vi "EC_Applied_Motion_SXSYSZ_20170419A_3chNoBKBACKUP.vi"() -> ()   [LabVIEW 2015]
uses:
  <vilib>/Instr/_visa.llb/VISA Configure Serial Port (Instr).vi
  <userlib>/caLab/Private/Put_DBL-1D_PV-1D.vi
  <userlib>/caLab/Private/Get_PV-1D.vi
  <vilib>/Utility/file.llb/Write To Spreadsheet File (I64).vi
  <vilib>/Utility/file.llb/Read From Spreadsheet File (I64).vi
panel:
  out "APX:FZ_DOWN":dbl
  out "APX:FZ_UP":dbl
  out "APX:FY_DOWN":dbl
  out "APX:FY_UP":dbl
  out "APX:FX_DOWN":dbl
  out "APX:FX_UP":dbl
  out "FZ Jog Counts In Range?":bool
  out "FY Jog Counts In Range?":bool
  out "FX Jog Counts In Range?":bool
  in  "FZ Jog counts":u8
  in  "FY Jog counts":u8
  in  "FX Jog counts":i8
  in  "GFS":bool=TRUE
  out "Isolated from GND?":bool
  in  "Crash Override":bool
  out "Dev5 Voltage 2":dbl
  out "Dev5 Voltage":dbl
  in  "Override":bool
  in  "APX:FZabs":dbl
  in  "Move Z":bool
  in  "Jog Z-":bool
  in  "Jog X-":bool
  in  "Jog Y-":bool
  out "Z Velocity MV mm/sec":dbl format="%.3f"
  out "Z Position MV mm":dbl
  out "Y Velocity MV mm/sec":dbl format="%.3f"
  out "Y Position MV mm":dbl
  out "X Velocity MV mm/sec":dbl format="%.3f"
  out "X Position MV mm":dbl
  in  "stop":bool
  in  "Tab Control 3":enum32{"Status", "Reset"}(tab)
  out "Y in Range":bool
  out "Y in Motion":bool
  out "X  in Range":bool
  out "X  in Motion":bool
  out "Z in Range":bool
  out "Z in Motion":bool
  out "X Ready":bool
  out "Y Ready":bool
  out "Z Ready":bool
  in  "Reset Y Position mm":dbl
  out "Reset Y Motor Steps":i32
  in  "Reset X Position mm":dbl
  out "Reset X Motor Steps":i32
  in  "Reset Z Position mm":dbl
  out "Reset Z Motor Steps":i32
  in  "Reset":bool
  in  "Tab Control":enum32{"mm", "preset", "step"}(tab)
  in  "APX:FXstep":dbl=0.1
  in  "FX Velocity SP mm/sec":dbl=0.01
  in  "APX:FYstep":dbl=0.05
  in  "FY Velocity SP mm/sec":dbl=0.01
  in  "APX:Fzstep":dbl=0.1
  in  "FZ Velocity SP mm/sec":dbl=0.01
  in  "Z Jog Set":bool
  in  "Y Jog Set":bool
  in  "X Jog Set":bool
  in  "X Velocity SP step/sec":i32 min=1 max=1000
  in  "Y Velocity SP step/sec":i32 min=1 max=1000
  in  "Z Velocity SP step/sec":i32 min=1 max=500
  in  "Y Step SP":i32=-20000 min=-800000 max=800000 step=500
  in  "X Step SP":i32=-20000 min=-750000 max=750000 step=500
  in  "Z Step SP":i32=-20000 min=-3000 max=102400000 step=500
  out "X Step PV":i32 max=2000
  out "Y Step PV":i32 max=2000
  out "Z Step PV":i32 max=2000
  out "R Step PV":i32 max=2000
  out "Z COM PORT":refnum<visa-resource-name>="COM5"
  out "Z Holding Current %":i32
  out "Z Run Current %":i32
  out "Z offset mm":dbl
  out "Z mm/rev":dbl
  out "Z steps/rev":u32
  out "Z  velocity PV step/sec":i32
  out "Z MINPOS":i32=-94296
  out "Z MAXPOS":i32=-34296
  in  "Jog Z+":bool
  out "Z Position mm PV":dbl
  out "X Position mm PV":dbl
  out "X velocity PV step/sec":i32
  in  "Jog X+":bool
  out "X Holding Current %":i32
  out "X Run Current %":i32
  out "X offset mm":dbl
  out "X mm/rev":dbl
  out "X steps/rev":u32
  out "X MAXPOS":i32=-34296
  out "X MINPOS":i32=-94296
  out "X COM PORT":refnum<visa-resource-name>="COM5"
  out "Y Holding Current %":i32
  out "Y Run Current %":i32
  out "Y Position mm PV":dbl
  out "Y offset mm":dbl
  out "Y mm/rev":dbl
  out "Y steps/rev":u32
  out "Y velocity PV step/sec":i32
  in  "Stop":bool
  in  "Jog Y+":bool
  out "Y MINPOS":i32=-94296
  out "Y MAXPOS":i32=-34296
  out "Y COM PORT":refnum<visa-resource-name>="COM5"
  # "APX:FY"
  # "x-ray"
  # "APX:FZ"
  # "APX:FX"
  # "SPEAR"
  # "APX:FinePos"
  # "Stage"
  # "Current position"
  # "Jog step/velovity"
  # "sample to SSRL"
  # "FX"
  # "FY"
  # "FZ"
  # "R,L = green"
  # "L"
  # "M"
  # "B"
  # "S"
  # "R"
  # "Preset position"
types:
  T1 = enum16{"Power-up Signature", "Accel Rate", "Accel Max", "Bit Rate", "Buffer Status", "Change Current", "Commence Jogging", "Change Jog Speed", "Continue", "Define Address", "Distance for FC,FM,FO,FY", "Decel Rate", "Distance or Position", "Define Limits", "Encoder Deadband", "Encoder Function", "Encoder Position", "Encoder Ratio", "Feed to Length with Speed Change", "Feed to Length", "Feed to Sensor with Mask Dist", "Feed to Length & Set Output", "Feed to Position", "Feed to Sensor", "Feed to Sensor w/safety", "Follow Handwheel", "Immediate Distance?", "Immediate Encoder?", "Immediate Low Output", "Immediate High Output", "Immediate Position?", "Input Status?", "Jog Accel/Decel", "Jog Disable", "Jog Enable", "Jog Speed", "Motor Disable", "Motor Enable", "Microstep Resolution", "Power up Current", "Power up Mode", "Pause", "Request Status", "Revision Level?", "Seek Home", "Stop Jogging", "Stop & Kill Buffer", "Set Output", "Set ABS Position", "Send String", "Stop", "Velocity for Speed Change", "Velocity Setting", "Wait for Input", "Wait Time"}
  T2 = enum8{"Enabled", "Disabled", "Disabled and Grayed Out"}
  T3 = cluster{"first row[0]":i64, "first row[1]":i64, "first row[2]":i64, "first row[3]":i64, "first row[4]":i64, "first row[5]":i64, "first row[6]":i64, "first row[7]":i64, "first row[8]":i64}
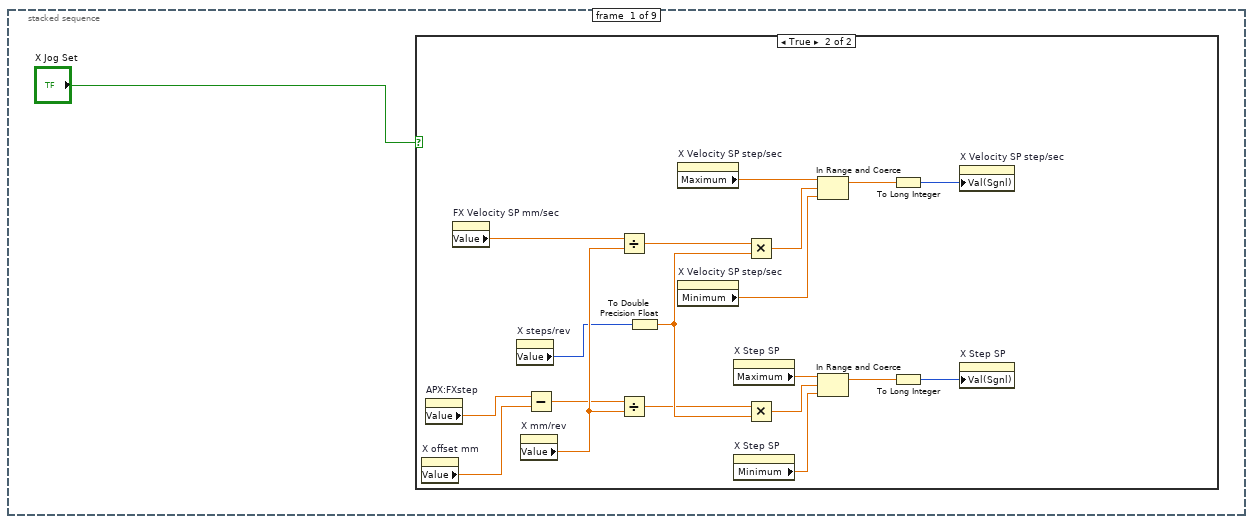
[diagram p5: hidden frame]
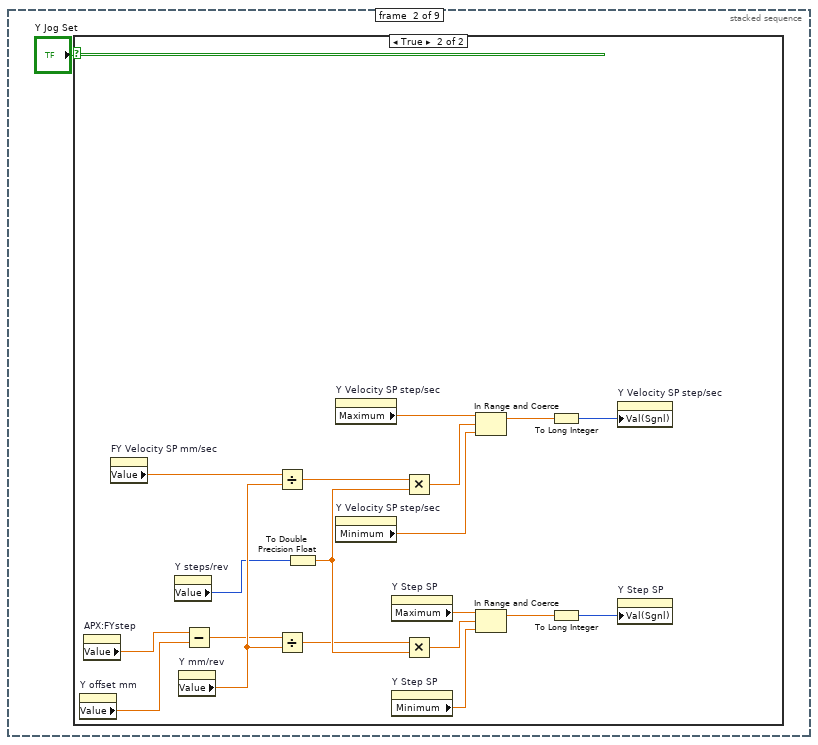
[diagram p7: hidden frame]
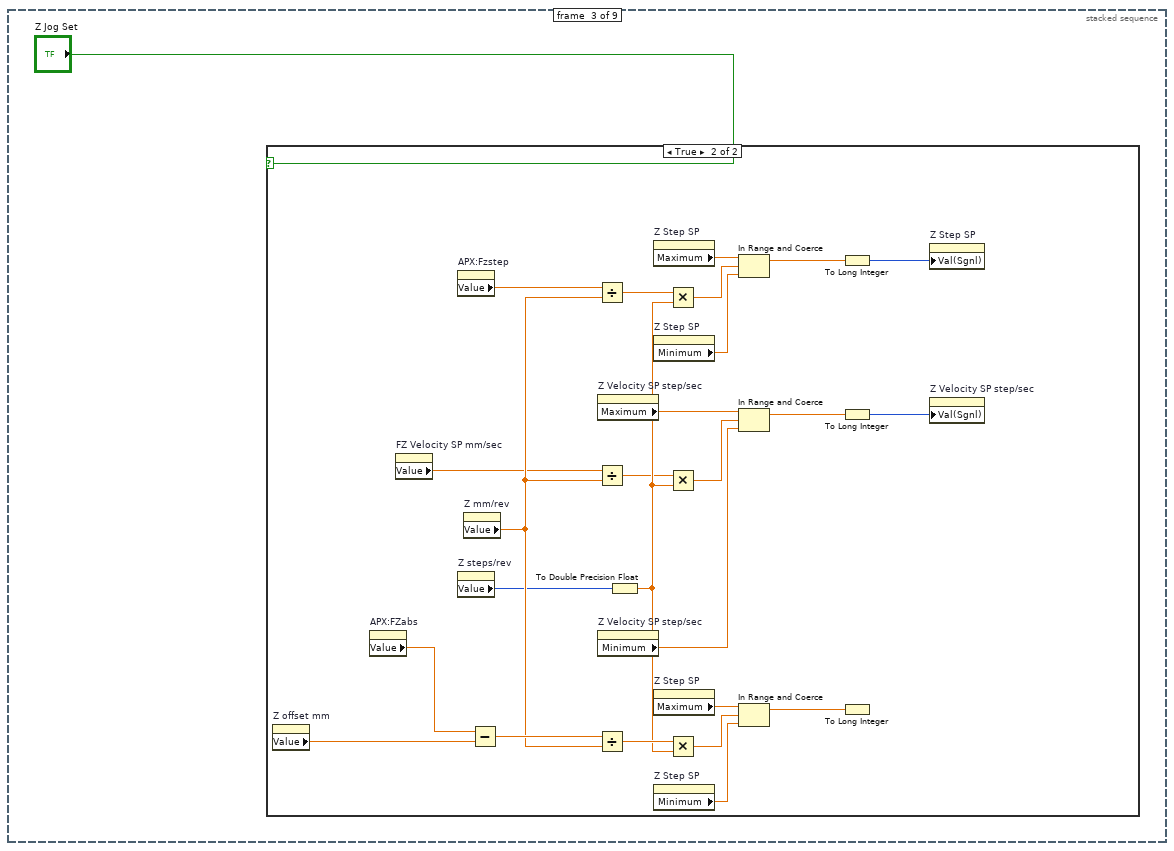
[diagram p9: hidden frame]
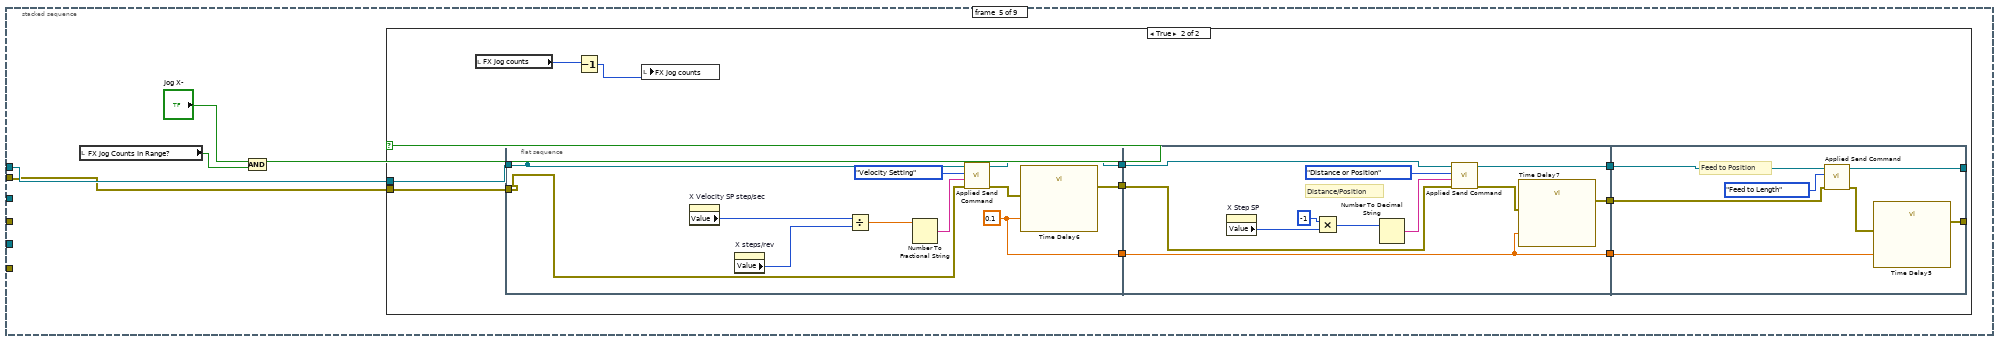
[diagram p12: hidden frame]
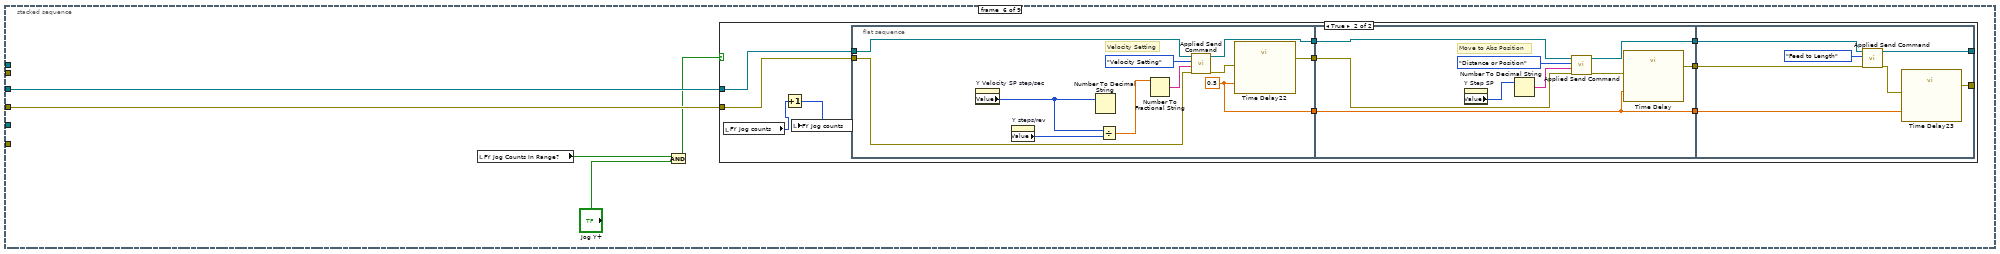
[diagram p14: hidden frame]
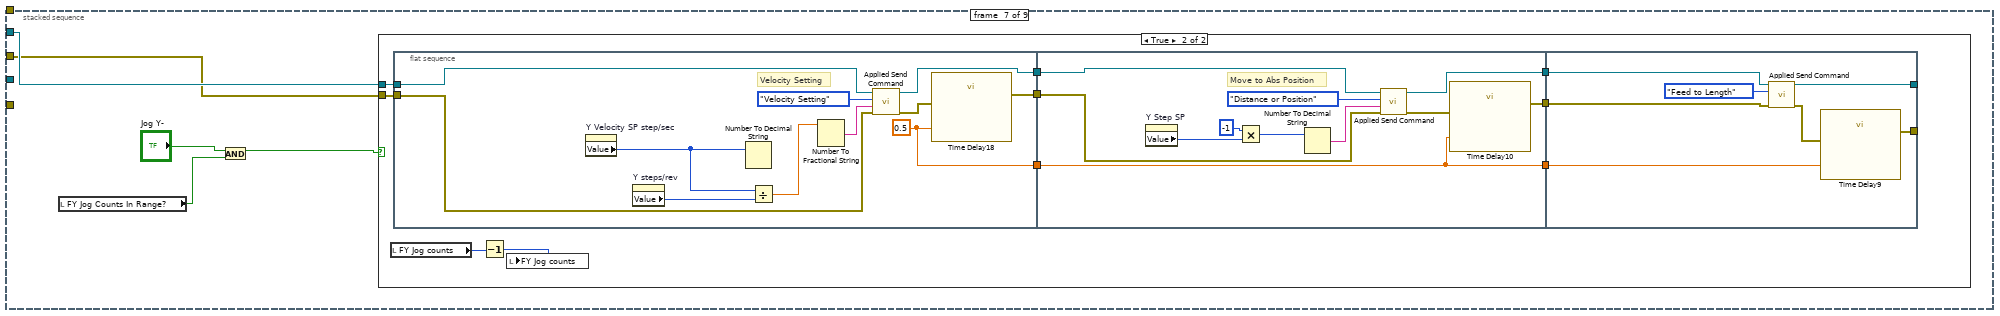
[diagram p16: hidden frame]
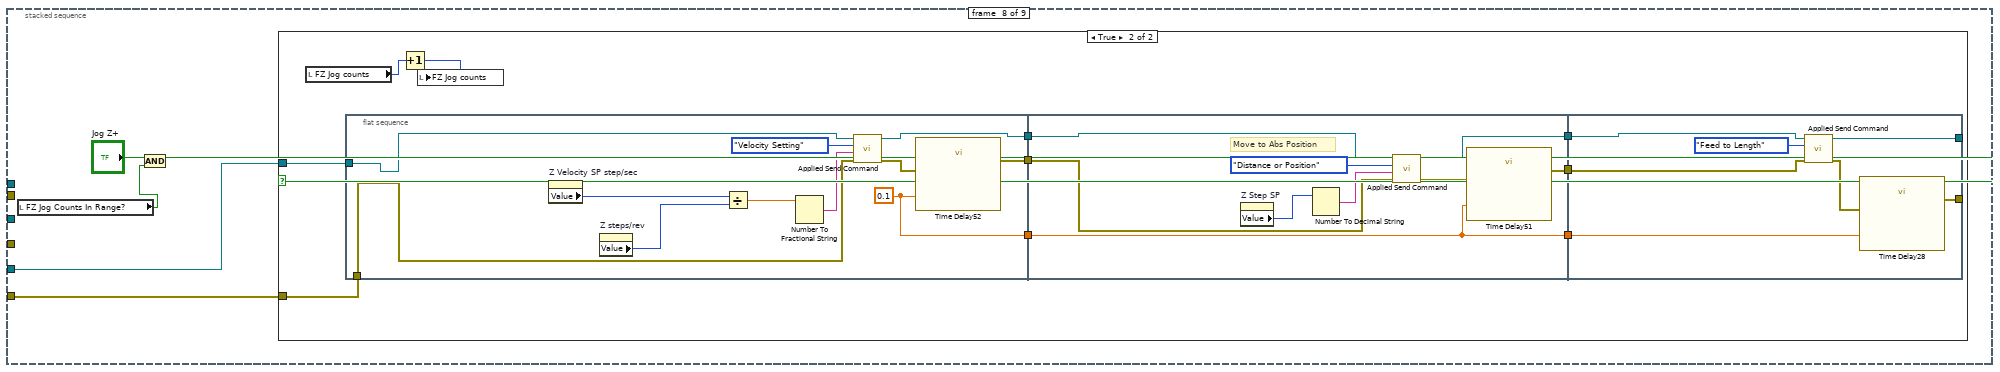
[diagram p18: hidden frame]
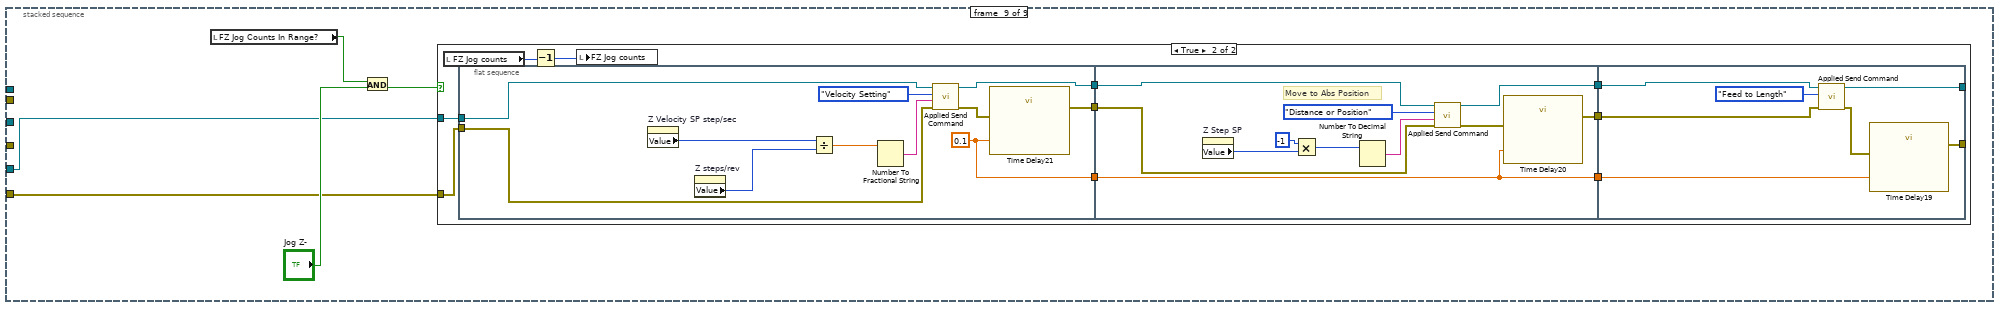
[diagram p20: hidden frame]
diagram:
  (unwired) FALSE
  n1 = flat-sequence {
    tunnel: [w58] -> w18
    tunnel: [w57] -> w17
    tunnel: w18 -> [w75]
    tunnel: w17 -> [w74]
    tunnel: [w73] -> w16
    tunnel: [w72] -> w15
    tunnel: [w78] -> w40
    tunnel: w16 -> [w86]
    tunnel: w15 -> [w85]
    tunnel: [w79] -> w14
    tunnel: w40 -> [w100]
    tunnel: [w99] -> w34
    tunnel: [w97] -> w33
    tunnel: [w102] -> w32
    tunnel: w14 -> [w101]
    tunnel: [w108] -> w38
    tunnel: [w109] -> w39
    tunnel: w34 -> [w109]
    tunnel: w33 -> [w108]
    tunnel: w32 -> [w107]
    frame #0 {
      "X Run Current %" <- 100 ("Run Current %")
      "X Holding Current %" <- 50 ("Holding Current %")
    }
    frame #1 {
      w45 = T2."Enabled" ("Disabled")
      n2 = property on="Jog X+" class="Bool"("DisabledEnum"=w45) -> ()  [unwired: 2 in, 2 out]
      n3 = property on="Jog X-" class="Bool"("DisabledEnum"=w45) -> ()  [unwired: 2 in, 2 out]
      n4 = property on="Jog Y+" class="Bool"("DisabledEnum"=w45) -> ()  [unwired: 2 in, 2 out]
      n5 = property on="Jog Z+" class="Bool"("DisabledEnum"=w45) -> ()  [unwired: 2 in, 2 out]
      n6 = property on="Jog Y-" class="Bool"("DisabledEnum"=w45) -> ()  [unwired: 2 in, 2 out]
      n7 = property on="Jog Z-" class="Bool"("DisabledEnum"=w45) -> ()  [unwired: 2 in, 2 out]
    }
    frame #2 {
      w48 = 0.21167 ("MM/rev")
      w51 = u32 20000 ("step/rev")
      w46 = 1000 ("Value (Signaling)")
      (unwired) 0.01 ("Value (Signaling)")
      n8 = property on="X Velocity SP step/sec" class="DigNum (strict)"("Minimum"=1.0 ("Data Entry Limits:Minimum")) -> ()  [unwired: 2 in, 2 out]
      n9 = property on="X Velocity SP step/sec" class="DigNum (strict)"("Val(Sgnl)"=w46) -> ()  [unwired: 2 in, 2 out]
      n10 = To Double Precision Float(number=w51) -> (double precision float=w50:dbl)
      n11 = To Double Precision Float(number=w46) -> (double precision float=w52:dbl)
      n12 = property on="X Velocity SP step/sec" class="DigNum (strict)"("Maximum"=w52) -> ()  [unwired: 2 in, 2 out]
      n13 = Divide(x=w52, y=w50) -> (x/y=w47:dbl)
      n14 = Multiply(x=w47, y=w48) -> (x*y=w49:dbl)
      n15 = property on="FX Velocity SP mm/sec" class="DigNum (strict)"("Val(Sgnl)"=w49) -> ()  [unwired: 2 in, 2 out]
      "X steps/rev" <- w51
      "X mm/rev" <- w48
    }
    frame #3 {
      w56 = -750000 ("lower limit")
      w55 = 750000 ("upper limit")
      n16 = property on="X Step SP" class="DigNum (strict)"("Maximum"=w55) -> ()  [unwired: 2 in, 2 out]
      n17 = property on="X Step SP" class="DigNum (strict)"("Minimum"=w56) -> ()  [unwired: 2 in, 2 out]
      "X offset mm" <- 0.0 ("offset")
      "X MAXPOS" <- w55
      "X MINPOS" <- w56
    }
    frame #4 {
      w65 = refnum<visa-resource-name> "COM21" ("COM PORT")
      w63 = u16 0 items=["None", "XON/XOFF", "RTS/CTS", "XON/XOFF & RTS/CTS", "DTR/DSR", "XON/XOFF & DTR/DSR"] ("flow control (0:none)")
      w62 = u16 10 items=["1.0"=10, "1.5"=15, "2.0"=20] ("stop bits (10: 1 bit)")
      # "Stop bits"
      n18 = call-poly "VISA Configure Serial Port"("VISA resource name"=w65, "timeout (10sec)"=u32 10000, "baud rate (9600)"=u32 9600, "data bits (8)"=u16 8, "parity (0:none)"=enum16{"None", "Odd", "Even", "Mark", "Space"}."None", "stop bits (10: 1 bit)"=w62, "flow control (0:none)"=w63) -> ("VISA resource name out"=w58:refnum<visa-resource-name>, "error out"=w57:errorcluster)  [unwired: 7 in]
      "X COM PORT" <- w65
    }
    frame #5 {
      n19 = property on="X Run Current" class="DigNum (strict)"() -> ("Value"=w70:i32)  [unwired: 2 in, 2 out]
      n20 = Divide(x=w70, y=100) -> (x/y=w67:dbl)
      n21 = Multiply(x=3.5 ("y"), y=w67) -> (x*y=w69:dbl)
      n22 = Number To Fractional String(number=w69) -> (F-format string=w71:string)  [unwired: 3 in]
      n23 = call "Applied Send Command.vi"("error in (no error)"=w74, "Extra"=w71, "Command"=T1."Change Current", "VISA resource name"=w75) -> ("error out"=w73:errorcluster, "VISA resource name out"=w72:refnum<visa-resource-name>)  [unwired: 3 in, 1 out]
    }
    frame #6 {
      # "VELOCITY"
      n24 = property on="X Velocity SP step/sec" class="DigNum (strict)"() -> ("Value"=w82:i32)  [unwired: 2 in, 2 out]
      n25 = property on="X steps/rev" class="DigNum (strict)"() -> ("Value"=w81:u32)  [unwired: 2 in, 2 out]
      n26 = Divide(x=w82, y=w81) -> (x/y=w80:dbl)
      n27 = Number To Fractional String(number=w80) -> (F-format string=w87:string)  [unwired: 3 in]
      n28 = call "Applied Send Command.vi"("error in (no error)"=w86, "Extra"=w87, "Command"=T1."Velocity Setting", "VISA resource name"=w85) -> ("error out"=w88:errorcluster, "VISA resource name out"=w95:refnum<visa-resource-name>)  [unwired: 3 in, 1 out]
      n29 = call "Time Delay30"("error in (no error)"=w88, "Delay Time (s)"=0.1) -> ("error out"=w93:errorcluster)  [unwired: 9 in]
      n30 = call "Applied Send Command.vi"("error in (no error)"=w93, "Extra"="", "Command"=T1."Velocity Setting", "VISA resource name"=w95) -> ("error out"=w78:errorcluster, "read buffer"=w91:string, "VISA resource name out"=w79:refnum<visa-resource-name>)  [unwired: 3 in]
      n31 = Fract/Exp String To Number(string=w91, offset=3) -> (number=w84:dbl)  [unwired: 2 in, 1 out]
      n32 = Multiply(x=w84, y=w81) -> (x*y=w83:dbl)
      n33 = property on="X velocity PV step/sec" class="DigNum (strict)"("Val(Sgnl)"=w83) -> ()  [unwired: 2 in, 2 out]
    }
    frame #7 {
      # "GET CURRENT POSITION"
      n34 = call "Applied Send Command.vi"("error in (no error)"=w100, "Extra"="", "Command"=T1."Immediate Position?", "VISA resource name"=w101) -> ("error out"=w98:errorcluster, "read buffer"=w104:string, "VISA resource name out"=w99:refnum<visa-resource-name>)  [unwired: 3 in]
      n35 = call "Time Delay13"("error in (no error)"=w98, "Delay Time (s)"=0.1) -> ("error out"=w97:errorcluster)  [unwired: 9 in]
      n36 = Hexadecimal String To Number(string=w104, offset=3) -> (number=w102:u32)  [unwired: 1 in, 1 out]
    }
    frame #8 {
      n37 = disable-structure shown="Disabled" {
        disable-tunnel: w107 -> [w110 _]
        frame Disabled {
          n38 = property on="X Step SP" class="DigNum (strict)"("Val(Sgnl)"=w110) -> ()  [unwired: 2 in, 2 out]
          n39 = property on="X Step SP" class="DigNum (strict)"() -> ("Maximum"=w113:dbl)  [unwired: 2 in, 2 out]
          n40 = property on="X Step SP" class="DigNum (strict)"() -> ("Minimum"=w112:dbl)  [unwired: 2 in, 2 out]
          n41 = In Range and Coerce(upper limit=w113, x=w110, lower limit=w112) -> (In Range?=w111:bool)  [unwired: 1 out]
          n42 = property on="X  in Range" class="Bool (strict)"("Val(Sgnl)"=w111) -> ()  [unwired: 2 in, 2 out]
        }
        frame Enabled {
        }
      }
    }
  }
  n43 = flat-sequence {
    frame #0 {
    }
    frame #1 {
      n44 = call-poly <vilib>:"Read From Spreadsheet File.vi"("file path (dialog if empty)"=path "S:/SSE/SCL2/POS.TXT") -> ("first row"=w114:i64[])  [unwired: 6 in, 4 out]
      n45 = Array To Cluster(array=w114) -> (cluster=w115:T3)
      n46 = Unbundle(w115) -> ("first row[0]"=w117:i64, "first row[1]"=w118:i64, "first row[2]"=w119:i64)  [unwired: 6 out]
      n47 = property on="Reset X Motor Steps" class="DigNum (strict)"("Val(Sgnl)"=w117) -> ()  [unwired: 2 in, 2 out]
      n48 = property on="Reset Y Motor Steps" class="DigNum (strict)"("Val(Sgnl)"=w118) -> ()  [unwired: 2 in, 2 out]
      n49 = property on="Reset Z Motor Steps" class="DigNum (strict)"("Val(Sgnl)"=w119) -> ()  [unwired: 2 in, 2 out]
    }
  }
  n50 = flat-sequence {
    tunnel: [w134] -> w5
    tunnel: [w133] -> w4
    tunnel: w5 -> [w148]
    tunnel: w4 -> [w147]
    tunnel: [w146] -> w3
    tunnel: [w145] -> w2
    tunnel: [w156] -> w31
    tunnel: [w155] -> w30
    tunnel: w3 -> [w158]
    tunnel: w2 -> [w157]
    tunnel: w31 -> [w173]
    tunnel: w30 -> [w172]
    tunnel: [w174] -> w29
    tunnel: [w175] -> w28
    tunnel: [w176] -> w1
    tunnel: [w184] -> w26
    tunnel: [w185] -> w27
    tunnel: w29 -> [w185]
    tunnel: w28 -> [w184]
    tunnel: w1 -> [w183]
    frame #0 {
      "Z Run Current %" <- 100 ("Z Run Current %")
      "Z Holding Current %" <- 50 ("Z Holding Current %")
    }
    frame #1 {
    }
    frame #2 {
      (unwired) 0.05 ("Value (Signaling)")
      w124 = 2.54 ("Z mm/rev")
      w123 = u32 20000 ("step/rev")
      w125 = 500 ("Value (Signaling)")
      n51 = property on="Z Velocity SP step/sec" class="DigNum (strict)"("Minimum"=1.0 ("Data Entry Limits:Minimum")) -> ()  [unwired: 2 in, 2 out]
      n52 = property on="Z Velocity SP step/sec" class="DigNum (strict)"("Val(Sgnl)"=w125) -> ()  [unwired: 2 in, 2 out]
      n53 = To Double Precision Float(number=w123) -> (double precision float=w128:dbl)
      n54 = To Double Precision Float(number=w125) -> (double precision float=w129:dbl)
      n55 = property on="Z Velocity SP step/sec" class="DigNum (strict)"("Maximum"=w129) -> ()  [unwired: 2 in, 2 out]
      n56 = Divide(x=w129, y=w128) -> (x/y=w126:dbl)
      n57 = Multiply(x=w126, y=w124) -> (x*y=w127:dbl)
      n58 = property on="FZ Velocity SP mm/sec" class="DigNum (strict)"("Val(Sgnl)"=w127) -> ()  [unwired: 2 in, 2 out]
      "Z mm/rev" <- w124
      "Z steps/rev" <- w123
    }
    frame #3 {
      w131 = -3000 ("lower limit")
      w130 = 102400000 ("upper limit")
      n59 = property on="Z Step SP" class="DigNum (strict)"("Minimum"=w131) -> ()  [unwired: 2 in, 2 out]
      n60 = property on="Z Step SP" class="DigNum (strict)"("Maximum"=w130) -> ()  [unwired: 2 in, 2 out]
      "Z offset mm" <- 0.0 ("Z offset mm")
      "Z MINPOS" <- w131
      "Z MAXPOS" <- w130
    }
    frame #4 {
      w141 = refnum<visa-resource-name> "COM23" ("COM PORT")
      w139 = u16 0 items=["None", "XON/XOFF", "RTS/CTS", "XON/XOFF & RTS/CTS", "DTR/DSR", "XON/XOFF & DTR/DSR"] ("flow control (0:none)")
      w138 = u16 10 items=["1.0"=10, "1.5"=15, "2.0"=20] ("stop bits (10: 1 bit)")
      # "Stop bits"
      n61 = call-poly "VISA Configure Serial Port"("VISA resource name"=w141, "timeout (10sec)"=u32 10000, "baud rate (9600)"=u32 9600, "data bits (8)"=u16 8, "parity (0:none)"=enum16{"None", "Odd", "Even", "Mark", "Space"}."None", "stop bits (10: 1 bit)"=w138, "flow control (0:none)"=w139) -> ("VISA resource name out"=w134:refnum<visa-resource-name>, "error out"=w133:errorcluster)  [unwired: 7 in]
      "Z COM PORT" <- w141
    }
    frame #5 {
      # "Run Current %"
      n62 = property on="Z Run Current %" class="DigNum (strict)"() -> ("Value"=w149:i32)  [unwired: 2 in, 2 out]
      n63 = Divide(x=w149, y=100) -> (x/y=w150:dbl)
      n64 = Multiply(x=w150, y=3.5) -> (x*y=w144:dbl)
      n65 = Number To Fractional String(number=w144) -> (F-format string=w151:string)  [unwired: 3 in]
      n66 = call "Applied Send Command.vi"("error in (no error)"=w147, "Extra"=w151, "Command"=T1."Change Current", "VISA resource name"=w148) -> ("error out"=w145:errorcluster, "VISA resource name out"=w146:refnum<visa-resource-name>)  [unwired: 3 in, 1 out]
    }
    frame #6 {
      # "VELOCITY"
      n67 = property on="Z Velocity SP step/sec" class="DigNum (strict)"() -> ("Value"=w153:i32)  [unwired: 2 in, 2 out]
      n68 = property on="Z steps/rev" class="DigNum (strict)"() -> ("Value"=w154:u32)  [unwired: 2 in, 2 out]
      n69 = Divide(x=w153, y=w154) -> (x/y=w161:dbl)
      n70 = Number To Fractional String(number=w161) -> (F-format string=w163:string)  [unwired: 3 in]
      n71 = call "Applied Send Command.vi"("error in (no error)"=w157, "Extra"=w163, "Command"=T1."Velocity Setting", "VISA resource name"=w158) -> ("error out"=w164:errorcluster, "VISA resource name out"=w171:refnum<visa-resource-name>)  [unwired: 3 in, 1 out]
      n72 = call "Time Delay2"("error in (no error)"=w164, "Delay Time (s)"=0.1) -> ("error out"=w169:errorcluster)  [unwired: 9 in]
      n73 = call "Applied Send Command.vi"("error in (no error)"=w169, "Extra"="", "Command"=T1."Velocity Setting", "VISA resource name"=w171) -> ("error out"=w155:errorcluster, "read buffer"=w167:string, "VISA resource name out"=w156:refnum<visa-resource-name>)  [unwired: 3 in]
      n74 = Fract/Exp String To Number(string=w167, offset=3) -> (number=w162:dbl)  [unwired: 2 in, 1 out]
      n75 = Multiply(x=w162, y=w154) -> (x*y=w159:dbl)
      n76 = property on="Z  velocity PV step/sec" class="DigNum (strict)"("Val(Sgnl)"=w159) -> ()  [unwired: 2 in, 2 out]
    }
    frame #7 {
      # "GET CURRENT POSITION"
      n77 = call "Applied Send Command.vi"("error in (no error)"=w172, "Extra"="", "Command"=T1."Immediate Position?", "VISA resource name"=w173) -> ("error out"=w178:errorcluster, "read buffer"=w180:string, "VISA resource name out"=w174:refnum<visa-resource-name>)  [unwired: 3 in]
      n78 = call "Time Delay8"("error in (no error)"=w178, "Delay Time (s)"=0.1) -> ("error out"=w175:errorcluster)  [unwired: 9 in]
      n79 = Hexadecimal String To Number(string=w180, offset=3) -> (number=w176:u32)  [unwired: 1 in, 1 out]
    }
    frame #8 {
      n80 = disable-structure shown="Disabled" {
        disable-tunnel: w183 -> [w188 _]
        frame Disabled {
          n81 = property on="Z Step SP" class="DigNum (strict)"("Val(Sgnl)"=w188) -> ()  [unwired: 2 in, 2 out]
          n82 = property on="Z Step SP" class="DigNum (strict)"() -> ("Maximum"=w187:dbl)  [unwired: 2 in, 2 out]
          n83 = property on="Z Step SP" class="DigNum (strict)"() -> ("Minimum"=w186:dbl)  [unwired: 2 in, 2 out]
          n84 = In Range and Coerce(upper limit=w187, x=w188, lower limit=w186) -> (In Range?=w189:bool)  [unwired: 1 out]
          n85 = property on="Z in Range" class="Bool (strict)"("Val(Sgnl)"=w189) -> ()  [unwired: 2 in, 2 out]
        }
        frame Enabled {
        }
      }
    }
  }
  n86 = flat-sequence {
    tunnel: [w204] -> w13
    tunnel: [w203] -> w12
    tunnel: w13 -> [w218]
    tunnel: w12 -> [w217]
    tunnel: [w216] -> w11
    tunnel: [w215] -> w10
    tunnel: w11 -> [w226]
    tunnel: w10 -> [w225]
    tunnel: [w224] -> w9
    tunnel: [w223] -> w8
    tunnel: [w243] -> w35
    tunnel: w9 -> [w246]
    tunnel: w8 -> [w245]
    tunnel: [w244] -> w7
    tunnel: [w242] -> w6
    tunnel: [w253] -> w41
    tunnel: [w255] -> w42
    tunnel: w35 -> [w253]
    tunnel: w7 -> [w255]
    tunnel: w6 -> [w254]
    frame #0 {
      "Y Run Current %" <- 100 ("Run Current %")
      "Y Holding Current %" <- 50 ("Holding Current %")
    }
    frame #1 {
    }
    frame #2 {
      w194 = 0.21167 ("MM/rev")
      w197 = u32 20000 ("step/rev")
      w192 = 1000 ("Value (Signaling)")
      (unwired) 0.01 ("Value (Signaling)")
      n87 = property on="Y Velocity SP step/sec" class="DigNum (strict)"("Minimum"=1.0 ("Data Entry Limits:Minimum")) -> ()  [unwired: 2 in, 2 out]
      n88 = property on="Y Velocity SP step/sec" class="DigNum (strict)"("Val(Sgnl)"=w192) -> ()  [unwired: 2 in, 2 out]
      n89 = To Double Precision Float(number=w197) -> (double precision float=w196:dbl)
      n90 = To Double Precision Float(number=w192) -> (double precision float=w198:dbl)
      n91 = property on="Y Velocity SP step/sec" class="DigNum (strict)"("Maximum"=w198) -> ()  [unwired: 2 in, 2 out]
      n92 = Divide(x=w198, y=w196) -> (x/y=w193:dbl)
      n93 = Multiply(x=w193, y=w194) -> (x*y=w195:dbl)
      n94 = property on="FY Velocity SP mm/sec" class="DigNum (strict)"("Val(Sgnl)"=w195) -> ()  [unwired: 2 in, 2 out]
      "Y steps/rev" <- w197
      "Y mm/rev" <- w194
    }
    frame #3 {
      w201 = -800000 ("lower limit")
      w202 = 800000 ("upper limit")
      n95 = property on="Y Step SP" class="DigNum (strict)"("Maximum"=w202) -> ()  [unwired: 2 in, 2 out]
      n96 = property on="Y Step SP" class="DigNum (strict)"("Minimum"=w201) -> ()  [unwired: 2 in, 2 out]
      "Y MAXPOS" <- w202
      "Y MINPOS" <- w201
      "Y offset mm" <- 0.0 ("offset")
    }
    frame #4 {
      w211 = refnum<visa-resource-name> "COM22" ("COM PORT")
      w209 = u16 0 items=["None", "XON/XOFF", "RTS/CTS", "XON/XOFF & RTS/CTS", "DTR/DSR", "XON/XOFF & DTR/DSR"] ("flow control (0:none)")
      w208 = u16 10 items=["1.0"=10, "1.5"=15, "2.0"=20] ("stop bits (10: 1 bit)")
      # "Stop bits"
      n97 = call-poly "VISA Configure Serial Port"("VISA resource name"=w211, "timeout (10sec)"=u32 10000, "baud rate (9600)"=u32 9600, "data bits (8)"=u16 8, "parity (0:none)"=enum16{"None", "Odd", "Even", "Mark", "Space"}."None", "stop bits (10: 1 bit)"=w208, "flow control (0:none)"=w209) -> ("VISA resource name out"=w204:refnum<visa-resource-name>, "error out"=w203:errorcluster)  [unwired: 7 in]
      "Y COM PORT" <- w211
    }
    frame #5 {
      n98 = property on="Y Run Current %" class="DigNum (strict)"() -> ("Value"=w219:i32)  [unwired: 2 in, 2 out]
      n99 = Divide(x=w219, y=100) -> (x/y=w220:dbl)
      n100 = Multiply(x=w220, y=3.5) -> (x*y=w214:dbl)
      n101 = Number To Fractional String(number=w214) -> (F-format string=w221:string)  [unwired: 3 in]
      n102 = call "Applied Send Command.vi"("error in (no error)"=w217, "Extra"=w221, "Command"=T1."Change Current", "VISA resource name"=w218) -> ("error out"=w215:errorcluster, "VISA resource name out"=w216:refnum<visa-resource-name>)  [unwired: 3 in, 1 out]
    }
    frame #6 {
      # "VELOCITY"
      n103 = property on="Y Velocity SP step/sec" class="DigNum (strict)"() -> ("Value"=w227:i32)  [unwired: 2 in, 2 out]
      n104 = property on="Y steps/rev" class="DigNum (strict)"() -> ("Value"=w230:u32)  [unwired: 2 in, 2 out]
      n105 = Divide(x=w227, y=w230) -> (x/y=w229:dbl)
      n106 = Number To Fractional String(number=w229) -> (F-format string=w233:string)  [unwired: 3 in]
      n107 = call "Applied Send Command.vi"("error in (no error)"=w225, "Extra"=w233, "Command"=T1."Velocity Setting", "VISA resource name"=w226) -> ("error out"=w234:errorcluster, "VISA resource name out"=w241:refnum<visa-resource-name>)  [unwired: 3 in, 1 out]
      n108 = call "Time Delay36"("error in (no error)"=w234, "Delay Time (s)"=0.1) -> ("error out"=w239:errorcluster)  [unwired: 9 in]
      n109 = call "Applied Send Command.vi"("error in (no error)"=w239, "Extra"="", "Command"=T1."Velocity Setting", "VISA resource name"=w241) -> ("error out"=w223:errorcluster, "read buffer"=w237:string, "VISA resource name out"=w224:refnum<visa-resource-name>)  [unwired: 3 in]
      n110 = Fract/Exp String To Number(string=w237, offset=3) -> (number=w232:dbl)  [unwired: 2 in, 1 out]
      n111 = Multiply(x=w232, y=w230) -> (x*y=w231:dbl)
      n112 = property on="Y velocity PV step/sec" class="DigNum (strict)"("Val(Sgnl)"=w231) -> ()  [unwired: 2 in, 2 out]
    }
    frame #7 {
      # "GET CURRENT POSITION"
      n113 = call "Applied Send Command.vi"("error in (no error)"=w245, "Extra"="", "Command"=T1."Immediate Position?", "VISA resource name"=w246) -> ("error out"=w248:errorcluster, "read buffer"=w250:string, "VISA resource name out"=w244:refnum<visa-resource-name>)  [unwired: 3 in]
      n114 = call "Time Delay37"("error in (no error)"=w248, "Delay Time (s)"=0.1) -> ("error out"=w243:errorcluster)  [unwired: 9 in]
      n115 = Hexadecimal String To Number(string=w250, offset=3) -> (number=w242:u32)  [unwired: 1 in, 1 out]
    }
    frame #8 {
      n116 = disable-structure shown="Disabled" {
        disable-tunnel: w254 -> [w258 _]
        frame Disabled {
          n117 = property on="Y Step SP" class="DigNum (strict)"("Val(Sgnl)"=w258) -> ()  [unwired: 2 in, 2 out]
          n118 = property on="Y Step SP" class="DigNum (strict)"() -> ("Maximum"=w257:dbl)  [unwired: 2 in, 2 out]
          n119 = property on="Y Step SP" class="DigNum (strict)"() -> ("Minimum"=w256:dbl)  [unwired: 2 in, 2 out]
          n120 = In Range and Coerce(upper limit=w257, x=w258, lower limit=w256) -> (In Range?=w259:bool)  [unwired: 1 out]
          n121 = property on="Y in Range" class="Bool (strict)"("Val(Sgnl)"=w259) -> ()  [unwired: 2 in, 2 out]
        }
        frame Enabled {
        }
      }
    }
  }
  n122 = while {
    tunnel: w42 -> [w275]
    tunnel: w41 -> [w274]
    tunnel: [w295] -> w22
    tunnel: [w294] -> w23
    tunnel: w39 -> [w277]
    tunnel: w38 -> [w276]
    tunnel: [w292] -> w37
    tunnel: [w291] -> w36
    tunnel: w27 -> [w273]
    tunnel: w26 -> [w272]
    tunnel: [w290] -> w25
    tunnel: [w289] -> w24
    tunnel: [w288] -> _
    tunnel: [w287] -> _
    stop <- "stop" stop-if-true
    n123 = flat-sequence {
      frame #0 {
      }
      frame #1 {
      }
    }
    n124 = flat-sequence {
      frame #0 {
      }
      frame #1 {
      }
    }
    n125 = local read "X Position mm PV"() -> (w284:dbl)
    n126 = local read "Y Position mm PV"() -> (w283:dbl)
    n127 = local read "Z Position mm PV"() -> (w285:dbl)
    n128 = local read "FZ Jog counts"() -> (w261:u8)
    n129 = local read "FY Jog counts"() -> (w265:u8)
    n130 = local read "FX Jog counts"() -> (w269:i8)
    n131 = Build Array("APX:PiezeX", "APX:PiezeY", "APX:PiezeZ") -> (w279:string[])
    n132 = Build Array(w284, w283, w285) -> (w278:dbl[])
    n133 = flat-sequence {
      frame #0 {
        n134 = disable-structure shown="Disabled" {
          frame Disabled {
            w662 = 10 ("number of samples")
            n135 = call "DAQ Assistant"("number of samples"=w662) -> ("data"=w667:dynamicdata)  [unwired: 16 in, 2 out]
            n136 = call "Convert from Dynamic Data"("Dynamic Data Type"=w667) -> ("Array"=w668:dbl[])  [unwired: 3 in]
            n137 = Add Array Elements(numeric array=w668) -> (sum=w666:dbl)
            n138 = Divide(x=w666, y=w662) -> (x/y=w665:dbl)
            n139 = Absolute Value(x=w665) -> (abs(x)=w669:dbl)
            "Dev5 Voltage" <- w669
            n140 = Multiply(x=0.5, y=0.8) -> (x*y=w663:dbl)
            n141 = Greater?(x=w669, y=w663) -> (0:w670:bool)
            n142 = case shown="True" "Override" {
              tunnel: [w672 TRUE] -> _
              tunnel: w670 -> [w672 _]
              frame False {
              }
              frame True {
              }
            }
          }
          frame Enabled {
          }
        }
      }
    }
    n143 = call-poly <userlib>:"CaLabPut.vi"("Values"=w278, "PV Names"=w279) -> ()  [unwired: 6 in, 4 out]
    n144 = In Range and Coerce(upper limit=10.0, x=w269, lower limit=-10.0) -> (In Range?=→"FX Jog Counts In Range?":bool)  [unwired: 1 out]
    n145 = In Range and Coerce(upper limit=4.0, x=w265, lower limit=-4.0) -> (In Range?=→"FY Jog Counts In Range?":bool)  [unwired: 1 out]
    n146 = In Range and Coerce(upper limit=20.0, x=w261, lower limit=-2.0) -> (In Range?=→"FZ Jog Counts In Range?":bool)  [unwired: 1 out]
    n147 = flat-sequence {
      frame #0 {
        w304 = 0 ("index (col)")
        w311 = 0.0 ("element")
        n148 = Build Array("APX:FX_UP", "APX:FX_DOWN", "APX:FY_UP", "APX:FY_DOWN", "APX:FZ_UP", "APX:FZ_DOWN") -> (w312:string[])
        n149 = call-poly "CaLabGet.vi"("PV Names"=w312) -> ("Value Array (number)"=w302:dbl[][])  [unwired: 8 in, 6 out]
        n150 = Build Array(w311, w311, w311, w311, w311, w311) -> (w310:dbl[])
        n151 = call-poly <userlib>:"CaLabPut.vi"("Values"=w310, "PV Names"=w312) -> ()  [unwired: 6 in, 4 out]
        n152 = Index Array(array=w302, index (row)=0 ("disabled index (row)"), index (col)=w304) -> (element=→"APX:FX_UP":dbl)
        n153 = Index Array(array=w302, index (row)=1, index (col)=w304) -> (element=→"APX:FX_DOWN":dbl)
        n154 = Index Array(array=w302, index (row)=4, index (col)=w304) -> (element=→"APX:FZ_UP":dbl)
        n155 = Index Array(array=w302, index (row)=2, index (col)=w304) -> (element=→"APX:FY_UP":dbl)
        n156 = Index Array(array=w302, index (row)=5, index (col)=w304) -> (element=→"APX:FZ_DOWN":dbl)
        n157 = Index Array(array=w302, index (row)=3, index (col)=w304) -> (element=→"APX:FY_DOWN":dbl)
      }
    }
    n158 = stacked-sequence {
      tunnel: w277 -> [_ _ _ w388 w430 _ _ _ _]
      tunnel: w276 -> [_ _ _ w387 w429 _ _ _ _]
      tunnel: w275 -> [_ _ _ _ _ w474 w517 _ _]
      tunnel: w274 -> [_ _ _ _ _ w473 w516 _ _]
      tunnel: w273 -> [_ _ _ _ _ _ _ w560 w602]
      tunnel: w272 -> [_ _ _ _ _ _ _ w559 w601]
      frame #0 {
        n159 = case shown="True" "X Jog Set" {
          frame False {
          }
          frame True {
            n160 = property on="X offset mm" class="DigNum (strict)"() -> ("Value"=w324:dbl)  [unwired: 2 in, 2 out]
            n161 = property on="APX:FXstep" class="DigNum (strict)"() -> ("Value"=w325:dbl)  [unwired: 2 in, 2 out]
            n162 = property on="FX Velocity SP mm/sec" class="DigNum (strict)"() -> ("Value"=w331:dbl)  [unwired: 2 in, 2 out]
            n163 = property on="X steps/rev" class="DigNum (strict)"() -> ("Value"=w322:u32)  [unwired: 2 in, 2 out]
            n164 = property on="X mm/rev" class="DigNum (strict)"() -> ("Value"=w338:dbl)  [unwired: 2 in, 2 out]
            n165 = Subtract(x=w325, y=w324) -> (x-y=w321:dbl)
            n166 = Divide(x=w331, y=w338) -> (x/y=w330:dbl)
            n167 = Divide(x=w321, y=w338) -> (x/y=w320:dbl)
            n168 = To Double Precision Float(number=w322) -> (double precision float=w337:dbl)
            n169 = property on="X Velocity SP step/sec" class="DigNum (strict)"() -> ("Maximum"=w335:dbl)  [unwired: 2 in, 2 out]
            n170 = property on="X Velocity SP step/sec" class="DigNum (strict)"() -> ("Minimum"=w336:dbl)  [unwired: 2 in, 2 out]
            n171 = property on="X Step SP" class="DigNum (strict)"() -> ("Maximum"=w328:dbl)  [unwired: 2 in, 2 out]
            n172 = property on="X Step SP" class="DigNum (strict)"() -> ("Minimum"=w329:dbl)  [unwired: 2 in, 2 out]
            n173 = Multiply(x=w330, y=w337) -> (x*y=w333:dbl)
            n174 = Multiply(x=w320, y=w337) -> (x*y=w326:dbl)
            n175 = In Range and Coerce(upper limit=w335, x=w333, lower limit=w336) -> (coerced(x)=w334:dbl)  [unwired: 1 out]
            n176 = In Range and Coerce(upper limit=w328, x=w326, lower limit=w329) -> (coerced(x)=w327:dbl)  [unwired: 1 out]
            n177 = To Long Integer(number=w334) -> (32bit integer=w332:i32)
            n178 = To Long Integer(number=w327) -> (32bit integer=w323:i32)
            n179 = property on="X Velocity SP step/sec" class="DigNum (strict)"("Val(Sgnl)"=w332) -> ()  [unwired: 2 in, 2 out]
            n180 = property on="X Step SP" class="DigNum (strict)"("Val(Sgnl)"=w323) -> ()  [unwired: 2 in, 2 out]
          }
        }
      }
      frame #1 {
        n181 = case shown="True" "Y Jog Set" {
          frame False {
          }
          frame True {
            n182 = property on="Y offset mm" class="DigNum (strict)"() -> ("Value"=w344:dbl)  [unwired: 2 in, 2 out]
            n183 = property on="APX:FYstep" class="DigNum (strict)"() -> ("Value"=w345:dbl)  [unwired: 2 in, 2 out]
            n184 = property on="FY Velocity SP mm/sec" class="DigNum (strict)"() -> ("Value"=w351:dbl)  [unwired: 2 in, 2 out]
            n185 = property on="Y steps/rev" class="DigNum (strict)"() -> ("Value"=w342:u32)  [unwired: 2 in, 2 out]
            n186 = property on="Y mm/rev" class="DigNum (strict)"() -> ("Value"=w358:dbl)  [unwired: 2 in, 2 out]
            n187 = Subtract(x=w345, y=w344) -> (x-y=w341:dbl)
            n188 = Divide(x=w351, y=w358) -> (x/y=w350:dbl)
            n189 = Divide(x=w341, y=w358) -> (x/y=w340:dbl)
            n190 = To Double Precision Float(number=w342) -> (double precision float=w357:dbl)
            n191 = property on="Y Velocity SP step/sec" class="DigNum (strict)"() -> ("Maximum"=w355:dbl)  [unwired: 2 in, 2 out]
            n192 = property on="Y Velocity SP step/sec" class="DigNum (strict)"() -> ("Minimum"=w356:dbl)  [unwired: 2 in, 2 out]
            n193 = property on="Y Step SP" class="DigNum (strict)"() -> ("Maximum"=w348:dbl)  [unwired: 2 in, 2 out]
            n194 = property on="Y Step SP" class="DigNum (strict)"() -> ("Minimum"=w349:dbl)  [unwired: 2 in, 2 out]
            n195 = Multiply(x=w350, y=w357) -> (x*y=w353:dbl)
            n196 = Multiply(x=w340, y=w357) -> (x*y=w346:dbl)
            n197 = In Range and Coerce(upper limit=w355, x=w353, lower limit=w356) -> (coerced(x)=w354:dbl)  [unwired: 1 out]
            n198 = In Range and Coerce(upper limit=w348, x=w346, lower limit=w349) -> (coerced(x)=w347:dbl)  [unwired: 1 out]
            n199 = To Long Integer(number=w354) -> (32bit integer=w352:i32)
            n200 = To Long Integer(number=w347) -> (32bit integer=w343:i32)
            n201 = property on="Y Velocity SP step/sec" class="DigNum (strict)"("Val(Sgnl)"=w352) -> ()  [unwired: 2 in, 2 out]
            n202 = property on="Y Step SP" class="DigNum (strict)"("Val(Sgnl)"=w343) -> ()  [unwired: 2 in, 2 out]
          }
        }
      }
      frame #2 {
        n203 = case shown="True" "Z Jog Set" {
          frame False {
          }
          frame True {
            n204 = property on="Z offset mm" class="DigNum (strict)"() -> ("Value"=w382:dbl)  [unwired: 2 in, 2 out]
            n205 = property on="APX:FZabs" class="DigNum (strict)"() -> ("Value"=w384:dbl)  [unwired: 2 in, 2 out]
            n206 = property on="FZ Velocity SP mm/sec" class="DigNum (strict)"() -> ("Value"=w369:dbl)  [unwired: 2 in, 2 out]
            n207 = property on="APX:Fzstep" class="DigNum (strict)"() -> ("Value"=w363:dbl)  [unwired: 2 in, 2 out]
            n208 = property on="Z steps/rev" class="DigNum (strict)"() -> ("Value"=w361:u32)  [unwired: 2 in, 2 out]
            n209 = property on="Z mm/rev" class="DigNum (strict)"() -> ("Value"=w381:dbl)  [unwired: 2 in, 2 out]
            n210 = Subtract(x=w384, y=w382) -> (x-y=w383:dbl)
            n211 = Divide(x=w363, y=w381) -> (x/y=w360:dbl)
            n212 = Divide(x=w369, y=w381) -> (x/y=w368:dbl)
            n213 = Divide(x=w383, y=w381) -> (x/y=w380:dbl)
            n214 = property on="Z Velocity SP step/sec" class="DigNum (strict)"() -> ("Maximum"=w373:dbl)  [unwired: 2 in, 2 out]
            n215 = property on="Z Velocity SP step/sec" class="DigNum (strict)"() -> ("Minimum"=w374:dbl)  [unwired: 2 in, 2 out]
            n216 = To Double Precision Float(number=w361) -> (double precision float=w379:dbl)
            n217 = property on="Z Step SP" class="DigNum (strict)"() -> ("Maximum"=w366:dbl)  [unwired: 2 in, 2 out]
            n218 = property on="Z Step SP" class="DigNum (strict)"() -> ("Minimum"=w367:dbl)  [unwired: 2 in, 2 out]
            n219 = property on="Z Step SP" class="DigNum (strict)"() -> ("Maximum"=w376:dbl)  [unwired: 2 in, 2 out]
            n220 = property on="Z Step SP" class="DigNum (strict)"() -> ("Minimum"=w377:dbl)  [unwired: 2 in, 2 out]
            n221 = Multiply(x=w360, y=w379) -> (x*y=w364:dbl)
            n222 = Multiply(x=w368, y=w379) -> (x*y=w371:dbl)
            n223 = Multiply(x=w380, y=w379) -> (x*y=w378:dbl)
            n224 = In Range and Coerce(upper limit=w366, x=w364, lower limit=w367) -> (coerced(x)=w365:dbl)  [unwired: 1 out]
            n225 = In Range and Coerce(upper limit=w373, x=w371, lower limit=w374) -> (coerced(x)=w372:dbl)  [unwired: 1 out]
            n226 = In Range and Coerce(upper limit=w376, x=w378, lower limit=w377) -> (coerced(x)=w375:dbl)  [unwired: 1 out]
            n227 = To Long Integer(number=w365) -> (32bit integer=w362:i32)
            n228 = To Long Integer(number=w372) -> (32bit integer=w370:i32)
            n229 = To Long Integer(number=w375) -> ()  [unwired: 1 out]
            n230 = property on="Z Step SP" class="DigNum (strict)"("Val(Sgnl)"=w362) -> ()  [unwired: 2 in, 2 out]
            n231 = property on="Z Velocity SP step/sec" class="DigNum (strict)"("Val(Sgnl)"=w370) -> ()  [unwired: 2 in, 2 out]
          }
        }
      }
      frame #3 {
        n232 = local read "FX Jog Counts In Range?"() -> (w385:bool)
        n233 = And(x="Jog X+", y=w385) -> (x .and. y?=w386:bool)
        n234 = case shown="True" w386 {
          tunnel: w388 -> [_ w393]
          tunnel: w387 -> [_ w392]
          frame False {
          }
          frame True {
            n235 = flat-sequence {
              tunnel: [w404] -> w399
              tunnel: [w401] -> w398
              tunnel: [w400] -> w397
              tunnel: w393 -> [w406]
              tunnel: w392 -> [w405]
              tunnel: w399 -> [w413]
              tunnel: [w412] -> w396
              tunnel: w398 -> [w414]
              tunnel: [w415] -> w395
              tunnel: w397 -> [w411]
              tunnel: [w411] -> w394
              tunnel: w396 -> [w426]
              tunnel: w395 -> [w425]
              tunnel: [w424] -> _
              tunnel: [w423] -> _
              tunnel: w394 -> [w422]
              frame #0 {
                w400 = 0.1 ("Delay Time (s)")
                n236 = property on="X Velocity SP step/sec" class="DigNum (strict)"() -> ("Value"=w403:i32)  [unwired: 2 in, 2 out]
                n237 = property on="X steps/rev" class="DigNum (strict)"() -> ("Value"=w407:u32)  [unwired: 2 in, 2 out]
                n238 = Divide(x=w403, y=w407) -> (x/y=w408:dbl)
                n239 = Number To Fractional String(number=w408) -> (F-format string=w409:string)  [unwired: 3 in]
                n240 = call "Applied Send Command.vi"("error in (no error)"=w405, "Extra"=w409, "Command"=T1."Velocity Setting", "VISA resource name"=w406) -> ("error out"=w402:errorcluster, "VISA resource name out"=w404:refnum<visa-resource-name>)  [unwired: 3 in, 1 out]
                n241 = call "Time Delay14"("error in (no error)"=w402, "Delay Time (s)"=w400) -> ("error out"=w401:errorcluster)  [unwired: 9 in]
              }
              frame #1 {
                # "Distance/Position"
                n242 = property on="X Step SP" class="DigNum (strict)"() -> ("Value"=w416:i32)  [unwired: 2 in, 2 out]
                n243 = Number To Decimal String(number=w416) -> (decimal integer string=w418:string)  [unwired: 1 in]
                n244 = call "Applied Send Command.vi"("error in (no error)"=w414, "Extra"=w418, "Command"=T1."Distance or Position", "VISA resource name"=w413) -> ("error out"=w417:errorcluster, "VISA resource name out"=w412:refnum<visa-resource-name>)  [unwired: 3 in, 1 out]
                n245 = call "Time Delay31"("error in (no error)"=w417, "Delay Time (s)"=w411) -> ("error out"=w415:errorcluster)  [unwired: 9 in]
              }
              frame #2 {
                # "Feed to Position"
                n246 = call "Applied Send Command.vi"("error in (no error)"=w425, "Command"=T1."Feed to Length", "VISA resource name"=w426) -> ("error out"=w420:errorcluster, "VISA resource name out"=w424:refnum<visa-resource-name>)  [unwired: 4 in, 1 out]
                n247 = call "Time Delay15"("error in (no error)"=w420, "Delay Time (s)"=w422) -> ("error out"=w423:errorcluster)  [unwired: 9 in]
              }
            }
            n248 = local read "FX Jog counts"() -> (w391:i8)
            n249 = Increment(x=w391) -> (x+1=w390:i8)
            n250 = local write "FX Jog counts"(w390) -> ()
          }
        }
      }
      frame #4 {
        n251 = local read "FX Jog Counts In Range?"() -> (w427:bool)
        n252 = And(x="Jog X-", y=w427) -> (x .and. y?=w428:bool)
        n253 = case shown="True" w428 {
          tunnel: w430 -> [_ w435]
          tunnel: w429 -> [_ w434]
          frame False {
          }
          frame True {
            n254 = local read "FX Jog counts"() -> (w433:i8)
            n255 = flat-sequence {
              tunnel: [w448] -> w441
              tunnel: [w445] -> w440
              tunnel: [w444] -> w439
              tunnel: [w443] -> _
              tunnel: w435 -> [w443]
              tunnel: w434 -> [w442]
              tunnel: w441 -> [w457]
              tunnel: [w456] -> w438
              tunnel: w440 -> [w458]
              tunnel: [w459] -> w437
              tunnel: w439 -> [w455]
              tunnel: [w455] -> w436
              tunnel: w438 -> [w470]
              tunnel: w437 -> [w469]
              tunnel: [w468] -> _
              tunnel: [w467] -> _
              tunnel: w436 -> [w466]
              frame #0 {
                w444 = 0.1 ("Delay Time (s)")
                n256 = property on="X Velocity SP step/sec" class="DigNum (strict)"() -> ("Value"=w447:i32)  [unwired: 2 in, 2 out]
                n257 = property on="X steps/rev" class="DigNum (strict)"() -> ("Value"=w449:u32)  [unwired: 2 in, 2 out]
                n258 = Divide(x=w447, y=w449) -> (x/y=w450:dbl)
                n259 = Number To Fractional String(number=w450) -> (F-format string=w451:string)  [unwired: 3 in]
                n260 = call "Applied Send Command.vi"("error in (no error)"=w442, "Extra"=w451, "Command"=T1."Velocity Setting", "VISA resource name"=w443) -> ("error out"=w446:errorcluster, "VISA resource name out"=w448:refnum<visa-resource-name>)  [unwired: 3 in, 1 out]
                n261 = call "Time Delay6"("error in (no error)"=w446, "Delay Time (s)"=w444) -> ("error out"=w445:errorcluster)  [unwired: 9 in]
              }
              frame #1 {
                # "Distance/Position"
                n262 = property on="X Step SP" class="DigNum (strict)"() -> ("Value"=w460:i32)  [unwired: 2 in, 2 out]
                n263 = Multiply(x=-1, y=w460) -> (x*y=w454:i32)
                n264 = Number To Decimal String(number=w454) -> (decimal integer string=w462:string)  [unwired: 1 in]
                n265 = call "Applied Send Command.vi"("error in (no error)"=w458, "Extra"=w462, "Command"=T1."Distance or Position", "VISA resource name"=w457) -> ("error out"=w461:errorcluster, "VISA resource name out"=w456:refnum<visa-resource-name>)  [unwired: 3 in, 1 out]
                n266 = call "Time Delay7"("error in (no error)"=w461, "Delay Time (s)"=w455) -> ("error out"=w459:errorcluster)  [unwired: 9 in]
              }
              frame #2 {
                # "Feed to Position"
                n267 = call "Applied Send Command.vi"("error in (no error)"=w469, "Command"=T1."Feed to Length", "VISA resource name"=w470) -> ("error out"=w464:errorcluster, "VISA resource name out"=w468:refnum<visa-resource-name>)  [unwired: 4 in, 1 out]
                n268 = call "Time Delay5"("error in (no error)"=w464, "Delay Time (s)"=w466) -> ("error out"=w467:errorcluster)  [unwired: 9 in]
              }
            }
            n269 = Decrement(x=w433) -> (x-1=w432:i8)
            n270 = local write "FX Jog counts"(w432) -> ()
          }
        }
      }
      frame #5 {
        n271 = local read "FY Jog Counts In Range?"() -> (w471:bool)
        n272 = And(x=w471, y="Jog Y+") -> (x .and. y?=w472:bool)
        n273 = case shown="True" w472 {
          tunnel: w474 -> [_ w479]
          tunnel: w473 -> [_ w478]
          frame False {
          }
          frame True {
            n274 = local read "FY Jog counts"() -> (w477:u8)
            n275 = Increment(x=w477) -> (x+1=w476:u8)
            n276 = local write "FY Jog counts"(w476) -> ()
            n277 = flat-sequence {
              tunnel: [w492] -> w485
              tunnel: [w487] -> w484
              tunnel: [w486] -> w483
              tunnel: w478 -> [w491]
              tunnel: w479 -> [w490]
              tunnel: [w503] -> w482
              tunnel: [w498] -> w481
              tunnel: w485 -> [w501]
              tunnel: w484 -> [w502]
              tunnel: w483 -> [w499]
              tunnel: [w499] -> w480
              tunnel: [w508] -> _
              tunnel: [w511] -> _
              tunnel: w482 -> [w510]
              tunnel: w481 -> [w509]
              tunnel: w480 -> [w512]
              frame #0 {
                w486 = 0.5 ("Delay Time (s)")
                # "Velocity Setting"
                n278 = property on="Y Velocity SP step/sec" class="DigNum (strict)"() -> ("Value"=w495:i32)  [unwired: 2 in, 2 out]
                n279 = property on="Y steps/rev" class="DigNum (strict)"() -> ("Value"=w494:u32)  [unwired: 2 in, 2 out]
                n280 = Number To Decimal String(number=w495) -> ()  [unwired: 1 in, 1 out]
                n281 = Divide(x=w495, y=w494) -> (x/y=w496:dbl)
                n282 = Number To Fractional String(number=w496) -> (F-format string=w489:string)  [unwired: 3 in]
                n283 = call "Applied Send Command.vi"("error in (no error)"=w491, "Extra"=w489, "Command"=T1."Velocity Setting", "VISA resource name"=w490) -> ("error out"=w488:errorcluster, "VISA resource name out"=w492:refnum<visa-resource-name>)  [unwired: 3 in, 1 out]
                n284 = call "Time Delay22"("error in (no error)"=w488, "Delay Time (s)"=w486) -> ("error out"=w487:errorcluster)  [unwired: 9 in]
              }
              frame #1 {
                # "Move to Abs Position"
                n285 = property on="Y Step SP" class="DigNum (strict)"() -> ("Value"=w505:i32)  [unwired: 2 in, 2 out]
                n286 = Number To Decimal String(number=w505) -> (decimal integer string=w500:string)  [unwired: 1 in]
                n287 = call "Applied Send Command.vi"("error in (no error)"=w502, "Extra"=w500, "Command"=T1."Distance or Position", "VISA resource name"=w501) -> ("error out"=w497:errorcluster, "VISA resource name out"=w503:refnum<visa-resource-name>)  [unwired: 3 in, 1 out]
                n288 = call "Time Delay"("error in (no error)"=w497, "Delay Time (s)"=w499) -> ("error out"=w498:errorcluster)  [unwired: 9 in]
              }
              frame #2 {
                n289 = call "Applied Send Command.vi"("error in (no error)"=w509, "Command"=T1."Feed to Length", "VISA resource name"=w510) -> ("error out"=w506:errorcluster, "VISA resource name out"=w511:refnum<visa-resource-name>)  [unwired: 4 in, 1 out]
                n290 = call "Time Delay23"("error in (no error)"=w506, "Delay Time (s)"=w512) -> ("error out"=w508:errorcluster)  [unwired: 9 in]
              }
            }
          }
        }
      }
      frame #6 {
        n291 = local read "FY Jog Counts In Range?"() -> (w513:bool)
        n292 = And(x="Jog Y-", y=w513) -> (x .and. y?=w514:bool)
        n293 = case shown="True" w514 {
          tunnel: w517 -> [_ w521]
          tunnel: w516 -> [_ w520]
          frame False {
          }
          frame True {
            n294 = local read "FY Jog counts"() -> (w519:u8)
            n295 = flat-sequence {
              tunnel: [w534] -> w527
              tunnel: [w529] -> w526
              tunnel: [w528] -> w525
              tunnel: w520 -> [w533]
              tunnel: w521 -> [w532]
              tunnel: [w547] -> w524
              tunnel: [w542] -> w523
              tunnel: w527 -> [w545]
              tunnel: w526 -> [w546]
              tunnel: w525 -> [w543]
              tunnel: [w543] -> w522
              tunnel: [w552] -> _
              tunnel: [w555] -> _
              tunnel: w524 -> [w554]
              tunnel: w523 -> [w553]
              tunnel: w522 -> [w556]
              frame #0 {
                w528 = 0.5 ("Delay Time (s)")
                # "Velocity Setting"
                n296 = property on="Y Velocity SP step/sec" class="DigNum (strict)"() -> ("Value"=w537:i32)  [unwired: 2 in, 2 out]
                n297 = property on="Y steps/rev" class="DigNum (strict)"() -> ("Value"=w536:u32)  [unwired: 2 in, 2 out]
                n298 = Number To Decimal String(number=w537) -> ()  [unwired: 1 in, 1 out]
                n299 = Divide(x=w537, y=w536) -> (x/y=w538:dbl)
                n300 = Number To Fractional String(number=w538) -> (F-format string=w531:string)  [unwired: 3 in]
                n301 = call "Applied Send Command.vi"("error in (no error)"=w533, "Extra"=w531, "Command"=T1."Velocity Setting", "VISA resource name"=w532) -> ("error out"=w530:errorcluster, "VISA resource name out"=w534:refnum<visa-resource-name>)  [unwired: 3 in, 1 out]
                n302 = call "Time Delay18"("error in (no error)"=w530, "Delay Time (s)"=w528) -> ("error out"=w529:errorcluster)  [unwired: 9 in]
              }
              frame #1 {
                # "Move to Abs Position"
                n303 = property on="Y Step SP" class="DigNum (strict)"() -> ("Value"=w549:i32)  [unwired: 2 in, 2 out]
                n304 = Multiply(x=-1, y=w549) -> (x*y=w540:i32)
                n305 = Number To Decimal String(number=w540) -> (decimal integer string=w544:string)  [unwired: 1 in]
                n306 = call "Applied Send Command.vi"("error in (no error)"=w546, "Extra"=w544, "Command"=T1."Distance or Position", "VISA resource name"=w545) -> ("error out"=w541:errorcluster, "VISA resource name out"=w547:refnum<visa-resource-name>)  [unwired: 3 in, 1 out]
                n307 = call "Time Delay10"("error in (no error)"=w541, "Delay Time (s)"=w543) -> ("error out"=w542:errorcluster)  [unwired: 9 in]
              }
              frame #2 {
                n308 = call "Applied Send Command.vi"("error in (no error)"=w553, "Command"=T1."Feed to Length", "VISA resource name"=w554) -> ("error out"=w550:errorcluster, "VISA resource name out"=w555:refnum<visa-resource-name>)  [unwired: 4 in, 1 out]
                n309 = call "Time Delay9"("error in (no error)"=w550, "Delay Time (s)"=w556) -> ("error out"=w552:errorcluster)  [unwired: 9 in]
              }
            }
            n310 = Decrement(x=w519) -> (x-1=w518:u8)
            n311 = local write "FY Jog counts"(w518) -> ()
          }
        }
      }
      frame #7 {
        n312 = local read "FZ Jog Counts In Range?"() -> (w557:bool)
        n313 = And(x="Jog Z+", y=w557) -> (x .and. y?=w558:bool)
        n314 = case shown="True" w558 {
          tunnel: w560 -> [_ w565]
          tunnel: w559 -> [_ w564]
          frame False {
          }
          frame True {
            n315 = local read "FZ Jog counts"() -> (w563:u8)
            n316 = flat-sequence {
              tunnel: [w577] -> w571
              tunnel: [w575] -> w570
              tunnel: [w574] -> w569
              tunnel: w565 -> [w573]
              tunnel: w564 -> [w572]
              tunnel: [w586] -> w568
              tunnel: [w585] -> w567
              tunnel: w571 -> [w587]
              tunnel: w570 -> [w589]
              tunnel: w569 -> [w583]
              tunnel: [w583] -> w566
              tunnel: [w598] -> _
              tunnel: [w595] -> _
              tunnel: w568 -> [w596]
              tunnel: w567 -> [w594]
              tunnel: w566 -> [w597]
              frame #0 {
                w574 = 0.1 ("Delay Time (s)")
                n317 = property on="Z Velocity SP step/sec" class="DigNum (strict)"() -> ("Value"=w579:i32)  [unwired: 2 in, 2 out]
                n318 = property on="Z steps/rev" class="DigNum (strict)"() -> ("Value"=w578:u32)  [unwired: 2 in, 2 out]
                n319 = Divide(x=w579, y=w578) -> (x/y=w580:dbl)
                n320 = Number To Fractional String(number=w580) -> (F-format string=w581:string)  [unwired: 3 in]
                n321 = call "Applied Send Command.vi"("error in (no error)"=w572, "Extra"=w581, "Command"=T1."Velocity Setting", "VISA resource name"=w573) -> ("error out"=w576:errorcluster, "VISA resource name out"=w577:refnum<visa-resource-name>)  [unwired: 3 in, 1 out]
                n322 = call "Time Delay52"("error in (no error)"=w576, "Delay Time (s)"=w574) -> ("error out"=w575:errorcluster)  [unwired: 9 in]
              }
              frame #1 {
                # "Move to Abs Position"
                n323 = property on="Z Step SP" class="DigNum (strict)"() -> ("Value"=w591:i32)  [unwired: 2 in, 2 out]
                n324 = Number To Decimal String(number=w591) -> (decimal integer string=w588:string)  [unwired: 1 in]
                n325 = call "Applied Send Command.vi"("error in (no error)"=w589, "Extra"=w588, "Command"=T1."Distance or Position", "VISA resource name"=w587) -> ("error out"=w584:errorcluster, "VISA resource name out"=w586:refnum<visa-resource-name>)  [unwired: 3 in, 1 out]
                n326 = call "Time Delay51"("error in (no error)"=w584, "Delay Time (s)"=w583) -> ("error out"=w585:errorcluster)  [unwired: 9 in]
              }
              frame #2 {
                n327 = call "Applied Send Command.vi"("error in (no error)"=w594, "Command"=T1."Feed to Length", "VISA resource name"=w596) -> ("error out"=w592:errorcluster, "VISA resource name out"=w595:refnum<visa-resource-name>)  [unwired: 4 in, 1 out]
                n328 = call "Time Delay28"("error in (no error)"=w592, "Delay Time (s)"=w597) -> ("error out"=w598:errorcluster)  [unwired: 9 in]
              }
            }
            n329 = Increment(x=w563) -> (x+1=w562:u8)
            n330 = local write "FZ Jog counts"(w562) -> ()
          }
        }
      }
      frame #8 {
        n331 = local read "FZ Jog Counts In Range?"() -> (w599:bool)
        n332 = And(x=w599, y="Jog Z-") -> (x .and. y?=w600:bool)
        n333 = case shown="True" w600 {
          tunnel: w602 -> [_ w607]
          tunnel: w601 -> [_ w606]
          frame False {
          }
          frame True {
            n334 = local read "FZ Jog counts"() -> (w605:u8)
            n335 = flat-sequence {
              tunnel: [w617] -> w613
              tunnel: [w615] -> w612
              tunnel: [w614] -> w611
              tunnel: w606 -> [w618]
              tunnel: w607 -> [w619]
              tunnel: [w630] -> w610
              tunnel: [w629] -> w609
              tunnel: w613 -> [w631]
              tunnel: w612 -> [w633]
              tunnel: w611 -> [w627]
              tunnel: [w627] -> w608
              tunnel: [w642] -> _
              tunnel: [w639] -> _
              tunnel: w610 -> [w640]
              tunnel: w609 -> [w638]
              tunnel: w608 -> [w641]
              frame #0 {
                w614 = 0.1 ("Delay Time (s)")
                n336 = property on="Z Velocity SP step/sec" class="DigNum (strict)"() -> ("Value"=w621:i32)  [unwired: 2 in, 2 out]
                n337 = property on="Z steps/rev" class="DigNum (strict)"() -> ("Value"=w620:u32)  [unwired: 2 in, 2 out]
                n338 = Divide(x=w621, y=w620) -> (x/y=w622:dbl)
                n339 = Number To Fractional String(number=w622) -> (F-format string=w623:string)  [unwired: 3 in]
                n340 = call "Applied Send Command.vi"("error in (no error)"=w618, "Extra"=w623, "Command"=T1."Velocity Setting", "VISA resource name"=w619) -> ("error out"=w616:errorcluster, "VISA resource name out"=w617:refnum<visa-resource-name>)  [unwired: 3 in, 1 out]
                n341 = call "Time Delay21"("error in (no error)"=w616, "Delay Time (s)"=w614) -> ("error out"=w615:errorcluster)  [unwired: 9 in]
              }
              frame #1 {
                # "Move to Abs Position"
                n342 = property on="Z Step SP" class="DigNum (strict)"() -> ("Value"=w635:i32)  [unwired: 2 in, 2 out]
                n343 = Multiply(x=-1, y=w635) -> (x*y=w626:i32)
                n344 = Number To Decimal String(number=w626) -> (decimal integer string=w632:string)  [unwired: 1 in]
                n345 = call "Applied Send Command.vi"("error in (no error)"=w633, "Extra"=w632, "Command"=T1."Distance or Position", "VISA resource name"=w631) -> ("error out"=w628:errorcluster, "VISA resource name out"=w630:refnum<visa-resource-name>)  [unwired: 3 in, 1 out]
                n346 = call "Time Delay20"("error in (no error)"=w628, "Delay Time (s)"=w627) -> ("error out"=w629:errorcluster)  [unwired: 9 in]
              }
              frame #2 {
                n347 = call "Applied Send Command.vi"("error in (no error)"=w638, "Command"=T1."Feed to Length", "VISA resource name"=w640) -> ("error out"=w636:errorcluster, "VISA resource name out"=w639:refnum<visa-resource-name>)  [unwired: 4 in, 1 out]
                n348 = call "Time Delay19"("error in (no error)"=w636, "Delay Time (s)"=w641) -> ("error out"=w642:errorcluster)  [unwired: 9 in]
              }
            }
            n349 = Decrement(x=w605) -> (x-1=w604:u8)
            n350 = local write "FZ Jog counts"(w604) -> ()
          }
        }
      }
    }
    n351 = event shown="[0] Timeout" {
      selector: _ -> [_ _ _ _ _ _]
      dyn-events: _ -> [_ _ _ _ _ _]
      timeout: 1 -> [_ _ _ _ _ _]
      tunnel: w274 -> [w735 _ _ w973 w985 w1012]
      tunnel: [_ _ _ w973 w983 w1010] -> w295
      tunnel: w275 -> [w707 _ _ w974 w986 w1013]
      tunnel: [_ _ _ w974 w984 w1011] -> w294
      tunnel: w277 -> [w706 _ _ _ w980 w1009]
      tunnel: w276 -> [w718 _ _ _ w979 w1008]
      tunnel: [_ _ _ _ w982 w1007] -> w292
      tunnel: [_ _ _ _ w981 w1006] -> w291
      tunnel: w273 -> [w708 _ _ _ w978 w1005]
      tunnel: w272 -> [w709 _ _ _ w977 w1004]
      tunnel: [_ _ _ _ w976 _] -> w290
      tunnel: [_ _ _ _ w975 _] -> w289
      tunnel: [_ _ _ _ _ w1003] -> w288
      tunnel: [_ _ _ _ _ w1002] -> w287
      event Timeout {
        n352 = event-data() -> ()  [unwired: 1 in, 2 out]
        n353 = flat-sequence {
          tunnel: [w747] -> w717
          tunnel: [w760] -> w716
          tunnel: [w769] -> w715
          tunnel: [w740] -> w714
          tunnel: w708 -> [w755]
          tunnel: w709 -> [w756]
          tunnel: [w738] -> w675
          tunnel: w717 -> [w779]
          tunnel: [w779] -> w713
          tunnel: w716 -> [w778]
          tunnel: [w778] -> w712
          tunnel: w715 -> [w777]
          tunnel: [w775] -> w711
          tunnel: w714 -> [w776]
          tunnel: [w776] -> w710
          tunnel: w713 -> [w782]
          tunnel: w712 -> [w783]
          tunnel: w711 -> [w781]
          tunnel: w710 -> [w780]
          tunnel: [w780] -> w683
          frame #0 {
            w759 = 0.5 ("Delay Time (s)")
            n354 = call "Applied Send Command.vi"("error in (no error)"=w756, "Command"=T1."Immediate Position?", "VISA resource name"=w755) -> ("error out"=w754:errorcluster, "read buffer"=w751:string, "VISA resource name out"=w749:refnum<visa-resource-name>)  [unwired: 4 in]
            n355 = Hexadecimal String To Number(string=w751, offset=3) -> (number=w752:u32)  [unwired: 1 in, 1 out]
            n356 = property on="Z Step SP" class="DigNum (strict)"() -> ("Maximum"=w771:dbl)  [unwired: 2 in, 2 out]
            n357 = property on="Z Step SP" class="DigNum (strict)"() -> ("Minimum"=w773:dbl)  [unwired: 2 in, 2 out]
            n358 = To Long Integer(number=w752) -> (32bit integer=w761:i32)
            n359 = property on="Z steps/rev" class="DigNum (strict)"() -> ("Value"=w767:u32)  [unwired: 2 in, 2 out]
            n360 = property on="Z Step PV" class="DigNum (strict)"("Val(Sgnl)"=w761) -> ()  [unwired: 2 in, 2 out]
            n361 = To Long Integer(number=w771) -> (32bit integer=w770:i32)
            n362 = To Long Integer(number=w773) -> (32bit integer=w772:i32)
            n363 = In Range and Coerce(upper limit=w770, x=w761, lower limit=w772) -> (In Range?=w769:bool)  [unwired: 1 out]
            n364 = To Double Precision Float(number=w761) -> (double precision float=w762:dbl)
            n365 = To Double Precision Float(number=w767) -> (double precision float=w768:dbl)
            n366 = property on="Z in Range" class="Bool (strict)"("Val(Sgnl)"=w769) -> ()  [unwired: 2 in, 2 out]
            n367 = Divide(x=w762, y=w768) -> (x/y=w766:dbl)
            n368 = call "Time Delay17"("error in (no error)"=w754, "Delay Time (s)"=w759) -> ("error out"=w739:errorcluster)  [unwired: 9 in]
            n369 = property on="Z mm/rev" class="DigNum (strict)"() -> ("Value"=w765:dbl)  [unwired: 2 in, 2 out]
            n370 = property on="Z offset mm" class="DigNum (strict)"() -> ("Value"=w763:dbl)  [unwired: 2 in, 2 out]
            n371 = Multiply(x=w766, y=w765) -> (x*y=w764:dbl)
            n372 = call "Applied Send Command.vi"("error in (no error)"=w739, "Command"=T1."Request Status", "VISA resource name"=w749) -> ("error out"=w748:errorcluster, "read buffer"=w744:string, "VISA resource name out"=w747:refnum<visa-resource-name>)  [unwired: 4 in]
            n373 = call "Time Delay16"("error in (no error)"=w748, "Delay Time (s)"=w759) -> ("error out"=w760:errorcluster)  [unwired: 9 in]
            n374 = Add(x=w764, y=w763) -> (x+y=w738:dbl)
            n375 = String Subset(string=w744, offset (0)=0, length (rest)=1 ("length (rest)")) -> (substring=w741:string)
            n376 = property on="Z Position mm PV" class="DigNum (strict)"("Val(Sgnl)"=w738) -> ()  [unwired: 2 in, 2 out]
            n377 = Equal?(x=w741, y="R") -> (x = y?=w758:bool)
            n378 = Not Equal?(x=w741, y="R") -> (x != y?=w740:bool)
            n379 = property on="Z Ready" class="Bool (strict)"("Val(Sgnl)"=w758) -> ()  [unwired: 2 in, 2 out]
            n380 = property on="Z in Motion" class="Bool (strict)"("Val(Sgnl)"=w740) -> ()  [unwired: 2 in, 2 out]
          }
          frame #1 {
            n381 = local read "Isolated from GND?"() -> (w774:bool)
            n382 = Or(x=w774, y=w777) -> (x .or. y?=w775:bool)
          }
          frame #2 {
            n383 = case shown="False" w781 {
              tunnel: w782 -> [w787 w790]
              tunnel: [w785 w790] -> _
              tunnel: [w784 w789] -> _
              tunnel: w783 -> [w786 w789]
              frame False {
                n384 = call "Applied Send Command.vi"("error in (no error)"=w786, "Command"=T1."Stop & Kill Buffer", "VISA resource name"=w787) -> ("error out"=w784:errorcluster, "VISA resource name out"=w785:refnum<visa-resource-name>)  [unwired: 4 in, 1 out]
              }
              frame True {
              }
            }
          }
        }
        n385 = property on="Y Step SP" class="DigNum (strict)"() -> ("Maximum"=w703:dbl)  [unwired: 2 in, 2 out]
        n386 = property on="Y Step SP" class="DigNum (strict)"() -> ("Minimum"=w702:dbl)  [unwired: 2 in, 2 out]
        n387 = property on="X Step SP" class="DigNum (strict)"() -> ("Maximum"=w698:dbl)  [unwired: 2 in, 2 out]
        n388 = property on="X Step SP" class="DigNum (strict)"() -> ("Minimum"=w699:dbl)  [unwired: 2 in, 2 out]
        n389 = Subtract(x=w703, y=w702) -> (x-y=w704:dbl)
        n390 = Subtract(x=w698, y=w699) -> (x-y=w700:dbl)
        n391 = property on="X Step PV" class="DigNum (strict)"() -> ("Value"=w697:i32)  [unwired: 2 in, 2 out]
        n392 = property on="Y Step PV" class="DigNum (strict)"() -> ("Value"=w696:i32)  [unwired: 2 in, 2 out]
        n393 = Divide(x=w704, y=2.0) -> (x/y=w692:dbl)
        n394 = Divide(x=w700, y=2.0) -> (x/y=w693:dbl)
        n395 = Absolute Value(x=w697) -> (abs(x)=w694:i32)
        n396 = Absolute Value(x=w696) -> (abs(x)=w695:i32)
        n397 = Absolute Value(x=w692) -> (abs(x)=w690:dbl)
        n398 = Absolute Value(x=w693) -> (abs(x)=w691:dbl)
        n399 = Multiply(x=w694, y=w695) -> (x*y=w689:i32)
        n400 = Multiply(x=w690, y=w691) -> (x*y=w688:dbl)
        n401 = Less Or Equal?(x=w689, y=w688) -> (x <= y?=w687:bool)
        n402 = flat-sequence {
          tunnel: w735 -> [w863]
          tunnel: w707 -> [w864]
          tunnel: [w860] -> w734
          tunnel: [w870] -> w732
          tunnel: [w849] -> w730
          tunnel: [w851] -> w728
          tunnel: w703 -> [w850]
          tunnel: w702 -> [w847]
          tunnel: w687 -> [w848]
          tunnel: [w846] -> w676
          tunnel: w734 -> [w889]
          tunnel: [w889] -> w733
          tunnel: w732 -> [w888]
          tunnel: [w888] -> w731
          tunnel: w730 -> [w887]
          tunnel: [w885] -> w729
          tunnel: w728 -> [w886]
          tunnel: [w886] -> w727
          tunnel: w733 -> [w892]
          tunnel: w731 -> [w893]
          tunnel: w729 -> [w891]
          tunnel: w727 -> [w890]
          tunnel: [w890] -> w684
          frame #0 {
            w869 = 0.5 ("Delay Time (s)")
            n403 = call "Applied Send Command.vi"("error in (no error)"=w863, "Command"=T1."Immediate Position?", "VISA resource name"=w864) -> ("error out"=w866:errorcluster, "read buffer"=w867:string, "VISA resource name out"=w861:refnum<visa-resource-name>)  [unwired: 4 in]
            n404 = To Long Integer(number=w850) -> (32bit integer=w881:i32)
            n405 = To Long Integer(number=w847) -> (32bit integer=w882:i32)
            n406 = Hexadecimal String To Number(string=w867, offset=3) -> (number=w871:u32)  [unwired: 1 in, 1 out]
            n407 = To Long Integer(number=w871) -> (32bit integer=w872:i32)
            n408 = property on="Y steps/rev" class="DigNum (strict)"() -> ("Value"=w878:u32)  [unwired: 2 in, 2 out]
            n409 = property on="Y Step PV" class="DigNum (strict)"("Val(Sgnl)"=w872) -> ()  [unwired: 2 in, 2 out]
            n410 = In Range and Coerce(upper limit=w881, x=w872, lower limit=w882) -> (In Range?=w880:bool)  [unwired: 1 out]
            n411 = To Double Precision Float(number=w872) -> (double precision float=w873:dbl)
            n412 = To Double Precision Float(number=w878) -> (double precision float=w879:dbl)
            n413 = Divide(x=w873, y=w879) -> (x/y=w877:dbl)
            n414 = And(x=w880, y=w848) -> (x .and. y?=w849:bool)
            n415 = property on="Y in Range" class="Bool (strict)"("Val(Sgnl)"=w849) -> ()  [unwired: 2 in, 2 out]
            n416 = call "Time Delay4"("error in (no error)"=w866, "Delay Time (s)"=w869) -> ("error out"=w859:errorcluster)  [unwired: 9 in]
            n417 = property on="Y mm/rev" class="DigNum (strict)"() -> ("Value"=w876:dbl)  [unwired: 2 in, 2 out]
            n418 = property on="Y offset mm" class="DigNum (strict)"() -> ("Value"=w874:dbl)  [unwired: 2 in, 2 out]
            n419 = Multiply(x=w877, y=w876) -> (x*y=w875:dbl)
            n420 = call "Applied Send Command.vi"("error in (no error)"=w859, "Command"=T1."Request Status", "VISA resource name"=w861) -> ("error out"=w858:errorcluster, "read buffer"=w855:string, "VISA resource name out"=w860:refnum<visa-resource-name>)  [unwired: 4 in]
            n421 = call "Time Delay3"("error in (no error)"=w858, "Delay Time (s)"=w869) -> ("error out"=w870:errorcluster)  [unwired: 9 in]
            n422 = Add(x=w875, y=w874) -> (x+y=w846:dbl)
            n423 = String Subset(string=w855, offset (0)=0, length (rest)=1 ("length (rest)")) -> (substring=w853:string)
            n424 = property on="Y Position mm PV" class="DigNum (strict)"("Val(Sgnl)"=w846) -> ()  [unwired: 2 in, 2 out]
            n425 = Equal?(x=w853, y="R") -> (x = y?=w868:bool)
            n426 = Not Equal?(x=w853, y="R") -> (x != y?=w851:bool)
            n427 = property on="Y Ready" class="Bool (strict)"("Val(Sgnl)"=w868) -> ()  [unwired: 2 in, 2 out]
            n428 = property on="Y in Motion" class="Bool (strict)"("Val(Sgnl)"=w851) -> ()  [unwired: 2 in, 2 out]
          }
          frame #1 {
            n429 = local read "Isolated from GND?"() -> (w884:bool)
            n430 = Or(x=w887, y=w884) -> (x .or. y?=w885:bool)
          }
          frame #2 {
            n431 = case shown="False" w891 {
              tunnel: w892 -> [w895 w900]
              tunnel: [w897 w900] -> _
              tunnel: [w896 w899] -> _
              tunnel: w893 -> [w894 w899]
              frame False {
                n432 = call "Applied Send Command.vi"("error in (no error)"=w894, "Command"=T1."Stop & Kill Buffer", "VISA resource name"=w895) -> ("error out"=w896:errorcluster, "VISA resource name out"=w897:refnum<visa-resource-name>)  [unwired: 4 in, 1 out]
              }
              frame True {
              }
            }
          }
        }
        n433 = flat-sequence {
          tunnel: [w804] -> w726
          tunnel: [w815] -> w725
          tunnel: [w793] -> w724
          tunnel: [w800] -> w723
          tunnel: w706 -> [w811]
          tunnel: w718 -> [w799]
          tunnel: w698 -> [w795]
          tunnel: w699 -> [w794]
          tunnel: w687 -> [w792]
          tunnel: [w791] -> w677
          tunnel: w726 -> [w834]
          tunnel: [w834] -> w722
          tunnel: w725 -> [w833]
          tunnel: [w833] -> w721
          tunnel: w724 -> [w830]
          tunnel: [w829] -> w720
          tunnel: w723 -> [w832]
          tunnel: [w832] -> w719
          tunnel: w722 -> [w838]
          tunnel: w721 -> [w837]
          tunnel: w720 -> [w836]
          tunnel: w719 -> [w835]
          tunnel: [w835] -> w685
          frame #0 {
            w814 = 0.5 ("Delay Time (s)")
            n434 = To Long Integer(number=w794) -> (32bit integer=w827:i32)
            n435 = To Long Integer(number=w795) -> (32bit integer=w826:i32)
            n436 = call "Applied Send Command.vi"("error in (no error)"=w799, "Command"=T1."Immediate Position?", "VISA resource name"=w811) -> ("error out"=w809:errorcluster, "read buffer"=w810:string, "VISA resource name out"=w805:refnum<visa-resource-name>)  [unwired: 4 in]
            n437 = Hexadecimal String To Number(string=w810, offset=3) -> (number=w816:u32)  [unwired: 1 in, 1 out]
            n438 = To Long Integer(number=w816) -> (32bit integer=w817:i32)
            n439 = property on="X steps/rev" class="DigNum (strict)"() -> ("Value"=w823:u32)  [unwired: 2 in, 2 out]
            n440 = property on="X Step PV" class="DigNum (strict)"("Val(Sgnl)"=w817) -> ()  [unwired: 2 in, 2 out]
            n441 = In Range and Coerce(upper limit=w826, x=w817, lower limit=w827) -> (In Range?=w825:bool)  [unwired: 1 out]
            n442 = To Double Precision Float(number=w817) -> (double precision float=w818:dbl)
            n443 = To Double Precision Float(number=w823) -> (double precision float=w824:dbl)
            n444 = Divide(x=w818, y=w824) -> (x/y=w822:dbl)
            n445 = And(x=w792, y=w825) -> (x .and. y?=w793:bool)
            n446 = property on="X  in Range" class="Bool (strict)"("Val(Sgnl)"=w793) -> ()  [unwired: 2 in, 2 out]
            n447 = call "Time Delay12"("error in (no error)"=w809, "Delay Time (s)"=w814) -> ("error out"=w802:errorcluster)  [unwired: 9 in]
            n448 = property on="X mm/rev" class="DigNum (strict)"() -> ("Value"=w821:dbl)  [unwired: 2 in, 2 out]
            n449 = property on="X offset mm" class="DigNum (strict)"() -> ("Value"=w819:dbl)  [unwired: 2 in, 2 out]
            n450 = Multiply(x=w822, y=w821) -> (x*y=w820:dbl)
            n451 = call "Applied Send Command.vi"("error in (no error)"=w802, "Command"=T1."Request Status", "VISA resource name"=w805) -> ("error out"=w803:errorcluster, "read buffer"=w807:string, "VISA resource name out"=w804:refnum<visa-resource-name>)  [unwired: 4 in]
            n452 = call "Time Delay11"("error in (no error)"=w803, "Delay Time (s)"=w814) -> ("error out"=w815:errorcluster)  [unwired: 9 in]
            n453 = Add(x=w820, y=w819) -> (x+y=w791:dbl)
            n454 = String Subset(string=w807, offset (0)=0, length (rest)=1 ("length (rest)")) -> (substring=w796:string)
            n455 = property on="X Position mm PV" class="DigNum (strict)"("Val(Sgnl)"=w791) -> ()  [unwired: 2 in, 2 out]
            n456 = Equal?(x=w796, y="R") -> (x = y?=w813:bool)
            n457 = Not Equal?(x=w796, y="R") -> (x != y?=w800:bool)
            n458 = property on="X Ready" class="Bool (strict)"("Val(Sgnl)"=w813) -> ()  [unwired: 2 in, 2 out]
            n459 = property on="X  in Motion" class="Bool (strict)"("Val(Sgnl)"=w800) -> ()  [unwired: 2 in, 2 out]
          }
          frame #1 {
            n460 = local read "Isolated from GND?"() -> (w831:bool)
            n461 = Or(x=w831, y=w830) -> (x .or. y?=w829:bool)
          }
          frame #2 {
            n462 = case shown="False" w836 {
              tunnel: w838 -> [w840 w845]
              tunnel: [w842 w845] -> _
              tunnel: [w843 w844] -> _
              tunnel: w837 -> [w839 w844]
              frame False {
                n463 = call "Applied Send Command.vi"("error in (no error)"=w839, "Command"=T1."Stop & Kill Buffer", "VISA resource name"=w840) -> ("error out"=w843:errorcluster, "VISA resource name out"=w842:refnum<visa-resource-name>)  [unwired: 4 in, 1 out]
              }
              frame True {
              }
            }
          }
        }
        n464 = Compound Arithmetic op=OR(w685, w684, w683) -> (w686:bool)
        n465 = case shown="False" w686 {
          tunnel: [T2."Enabled" ("Disabled") T2."Disabled and Grayed Out" ("Disabled")] -> w682
          frame False {
          }
          frame True {
          }
        }
        n466 = Build Array("APX:PiezoX", "APX:PiezoY", "APX:PiezoZ") -> (w681:string[])
        n467 = Build Array(w677, w676, w675) -> (w674:dbl[])
        n468 = call-poly <userlib>:"CaLabPut.vi"("Values"=w674, "PV Names"=w681) -> ()  [unwired: 6 in, 4 out]
        n469 = property on="Jog X-" class="Bool"("DisabledEnum"=w682) -> ()  [unwired: 2 in, 2 out]
        n470 = property on="Jog X+" class="Bool"("DisabledEnum"=w682) -> ()  [unwired: 2 in, 2 out]
        n471 = property on="Jog Y+" class="Bool"("DisabledEnum"=w682) -> ()  [unwired: 2 in, 2 out]
        n472 = property on="Jog Z+" class="Bool"("DisabledEnum"=w682) -> ()  [unwired: 2 in, 2 out]
        n473 = property on="Jog Y-" class="Bool"("DisabledEnum"=w682) -> ()  [unwired: 2 in, 2 out]
        n474 = property on="Jog Z-" class="Bool"("DisabledEnum"=w682) -> ()  [unwired: 2 in, 2 out]
      }
      event "Reset Y Position mm", "Reset X Position mm", "Reset Z Position mm": Value Change {
        n475 = event-data() -> ()  [unwired: 1 in, 5 out]
        n476 = property on="Reset Y Position mm" class="DigNum (strict)"() -> ("Value"=w927:dbl)  [unwired: 2 in, 2 out]
        n477 = property on="Reset X Position mm" class="DigNum (strict)"() -> ("Value"=w918:dbl)  [unwired: 2 in, 2 out]
        n478 = property on="Reset Z Position mm" class="DigNum (strict)"() -> ("Value"=w909:dbl)  [unwired: 2 in, 2 out]
        n479 = property on="Y offset mm" class="DigNum (strict)"() -> ("Value"=w919:dbl)  [unwired: 2 in, 2 out]
        n480 = property on="X offset mm" class="DigNum (strict)"() -> ("Value"=w910:dbl)  [unwired: 2 in, 2 out]
        n481 = property on="Z offset mm" class="DigNum (strict)"() -> ("Value"=w901:dbl)  [unwired: 2 in, 2 out]
        n482 = Subtract(x=w927, y=w919) -> (x-y=w926:dbl)
        n483 = Subtract(x=w918, y=w910) -> (x-y=w917:dbl)
        n484 = Subtract(x=w909, y=w901) -> (x-y=w908:dbl)
        n485 = property on="Y steps/rev" class="DigNum (strict)"() -> ("Value"=w921:u32)  [unwired: 2 in, 2 out]
        n486 = property on="X steps/rev" class="DigNum (strict)"() -> ("Value"=w912:u32)  [unwired: 2 in, 2 out]
        n487 = property on="Z steps/rev" class="DigNum (strict)"() -> ("Value"=w903:u32)  [unwired: 2 in, 2 out]
        n488 = property on="Y mm/rev" class="DigNum (strict)"() -> ("Value"=w920:dbl)  [unwired: 2 in, 2 out]
        n489 = property on="X mm/rev" class="DigNum (strict)"() -> ("Value"=w911:dbl)  [unwired: 2 in, 2 out]
        n490 = property on="Z mm/rev" class="DigNum (strict)"() -> ("Value"=w902:dbl)  [unwired: 2 in, 2 out]
        n491 = Divide(x=w926, y=w920) -> (x/y=w925:dbl)
        n492 = Divide(x=w917, y=w911) -> (x/y=w916:dbl)
        n493 = Divide(x=w908, y=w902) -> (x/y=w907:dbl)
        n494 = To Double Precision Float(number=w921) -> (double precision float=w924:dbl)
        n495 = To Double Precision Float(number=w912) -> (double precision float=w915:dbl)
        n496 = To Double Precision Float(number=w903) -> (double precision float=w906:dbl)
        n497 = Multiply(x=w925, y=w924) -> (x*y=w923:dbl)
        n498 = Multiply(x=w916, y=w915) -> (x*y=w914:dbl)
        n499 = Multiply(x=w907, y=w906) -> (x*y=w905:dbl)
        n500 = To Long Integer(number=w923) -> (32bit integer=w922:i32)
        n501 = To Long Integer(number=w914) -> (32bit integer=w913:i32)
        n502 = To Long Integer(number=w905) -> (32bit integer=w904:i32)
        n503 = property on="Reset Y Motor Steps" class="DigNum (strict)"("Val(Sgnl)"=w922) -> ()  [unwired: 2 in, 2 out]
        n504 = property on="Reset X Motor Steps" class="DigNum (strict)"("Val(Sgnl)"=w913) -> ()  [unwired: 2 in, 2 out]
        n505 = property on="Reset Z Motor Steps" class="DigNum (strict)"("Val(Sgnl)"=w904) -> ()  [unwired: 2 in, 2 out]
      }
      event "Y Velocity SP step/sec", "X Velocity SP step/sec", "Z Velocity SP step/sec", "Y Step SP", "X Step SP", "Z Step SP": Value Change {
        n506 = event-data() -> ()  [unwired: 1 in, 5 out]
        n507 = property on="X Velocity SP step/sec" class="DigNum (strict)"() -> ("Value"=w963:i32)  [unwired: 2 in, 2 out]
        n508 = property on="Y Velocity SP step/sec" class="DigNum (strict)"() -> ("Value"=w969:i32)  [unwired: 2 in, 2 out]
        n509 = property on="Z Velocity SP step/sec" class="DigNum (strict)"() -> ("Value"=w957:i32)  [unwired: 2 in, 2 out]
        n510 = property on="X steps/rev" class="DigNum (strict)"() -> ("Value"=w940:u32)  [unwired: 2 in, 2 out]
        n511 = property on="X steps/rev" class="DigNum (strict)"() -> ("Value"=w961:u32)  [unwired: 2 in, 2 out]
        n512 = property on="Y steps/rev" class="DigNum (strict)"() -> ("Value"=w948:u32)  [unwired: 2 in, 2 out]
        n513 = property on="Y steps/rev" class="DigNum (strict)"() -> ("Value"=w967:u32)  [unwired: 2 in, 2 out]
        n514 = property on="Z steps/rev" class="DigNum (strict)"() -> ("Value"=w932:u32)  [unwired: 2 in, 2 out]
        n515 = property on="Z steps/rev" class="DigNum (strict)"() -> ("Value"=w955:u32)  [unwired: 2 in, 2 out]
        n516 = property on="X Step SP" class="DigNum (strict)"() -> ("Value"=w942:i32)  [unwired: 2 in, 2 out]
        n517 = property on="Y Step SP" class="DigNum (strict)"() -> ("Value"=w950:i32)  [unwired: 2 in, 2 out]
        n518 = property on="Z Step SP" class="DigNum (strict)"() -> ("Value"=w934:i32)  [unwired: 2 in, 2 out]
        n519 = To Double Precision Float(number=w942) -> (double precision float=w943:dbl)
        n520 = To Double Precision Float(number=w940) -> (double precision float=w946:dbl)
        n521 = To Double Precision Float(number=w963) -> (double precision float=w964:dbl)
        n522 = To Double Precision Float(number=w961) -> (double precision float=w966:dbl)
        n523 = To Double Precision Float(number=w950) -> (double precision float=w951:dbl)
        n524 = To Double Precision Float(number=w948) -> (double precision float=w954:dbl)
        n525 = To Double Precision Float(number=w969) -> (double precision float=w970:dbl)
        n526 = To Double Precision Float(number=w967) -> (double precision float=w972:dbl)
        n527 = To Double Precision Float(number=w934) -> (double precision float=w935:dbl)
        n528 = To Double Precision Float(number=w932) -> (double precision float=w938:dbl)
        n529 = To Double Precision Float(number=w957) -> (double precision float=w958:dbl)
        n530 = To Double Precision Float(number=w955) -> (double precision float=w960:dbl)
        n531 = property on="X mm/rev" class="DigNum (strict)"() -> ("Value"=w929:dbl)  [unwired: 2 in, 2 out]
        n532 = property on="Y mm/rev" class="DigNum (strict)"() -> ("Value"=w928:dbl)  [unwired: 2 in, 2 out]
        n533 = property on="Z mm/rev" class="DigNum (strict)"() -> ("Value"=w930:dbl)  [unwired: 2 in, 2 out]
        n534 = Divide(x=w943, y=w946) -> (x/y=w945:dbl)
        n535 = Divide(x=w964, y=w966) -> (x/y=w965:dbl)
        n536 = Divide(x=w951, y=w954) -> (x/y=w953:dbl)
        n537 = Divide(x=w970, y=w972) -> (x/y=w971:dbl)
        n538 = Divide(x=w935, y=w938) -> (x/y=w937:dbl)
        n539 = Divide(x=w958, y=w960) -> (x/y=w959:dbl)
        n540 = property on="X offset mm" class="DigNum (strict)"() -> ("Value"=w939:dbl)  [unwired: 2 in, 2 out]
        n541 = property on="Y offset mm" class="DigNum (strict)"() -> ("Value"=w947:dbl)  [unwired: 2 in, 2 out]
        n542 = property on="Z offset mm" class="DigNum (strict)"() -> ("Value"=w931:dbl)  [unwired: 2 in, 2 out]
        n543 = Multiply(x=w945, y=w929) -> (x*y=w944:dbl)
        n544 = Multiply(x=w965, y=w929) -> (x*y=w962:dbl)
        n545 = Multiply(x=w953, y=w928) -> (x*y=w952:dbl)
        n546 = Multiply(x=w971, y=w928) -> (x*y=w968:dbl)
        n547 = Multiply(x=w937, y=w930) -> (x*y=w936:dbl)
        n548 = Multiply(x=w959, y=w930) -> (x*y=w956:dbl)
        n549 = property on="X Velocity MV mm/sec" class="DigNum (strict)"("Val(Sgnl)"=w962) -> ()  [unwired: 2 in, 2 out]
        n550 = property on="Y Velocity MV mm/sec" class="DigNum (strict)"("Val(Sgnl)"=w968) -> ()  [unwired: 2 in, 2 out]
        n551 = property on="Z Velocity MV mm/sec" class="DigNum (strict)"("Val(Sgnl)"=w956) -> ()  [unwired: 2 in, 2 out]
        n552 = Add(x=w944, y=w939) -> (x+y=w941:dbl)
        n553 = Add(x=w952, y=w947) -> (x+y=w949:dbl)
        n554 = Add(x=w936, y=w931) -> (x+y=w933:dbl)
        n555 = property on="X Position MV mm" class="DigNum (strict)"("Val(Sgnl)"=w941) -> ()  [unwired: 2 in, 2 out]
        n556 = property on="Y Position MV mm" class="DigNum (strict)"("Val(Sgnl)"=w949) -> ()  [unwired: 2 in, 2 out]
        n557 = property on="Z Position MV mm" class="DigNum (strict)"("Val(Sgnl)"=w933) -> ()  [unwired: 2 in, 2 out]
      }
      event Application Instance Close? {
        n558 = event-data() -> ()  [unwired: 1 in, 4 out]
        n559 = event-data() -> ()  [unwired: 3 in, 1 out]
      }
      event "Stop": Mouse Down {
        n560 = event-data() -> ()  [unwired: 1 in, 7 out]
        n561 = flat-sequence {
          tunnel: [w994] -> w982
          tunnel: [w993] -> w981
          tunnel: w980 -> [w995]
          tunnel: w979 -> [w992]
          frame #0 {
            n562 = call "Applied Send Command.vi"("error in (no error)"=w992, "Command"=T1."Stop", "VISA resource name"=w995) -> ("error out"=w993:errorcluster, "VISA resource name out"=w994:refnum<visa-resource-name>)  [unwired: 4 in, 1 out]
          }
        }
        n563 = flat-sequence {
          tunnel: w986 -> [w998]
          tunnel: w985 -> [w997]
          tunnel: [w999] -> w984
          tunnel: [w1000] -> w983
          frame #0 {
            n564 = call "Applied Send Command.vi"("error in (no error)"=w997, "Command"=T1."Stop", "VISA resource name"=w998) -> ("error out"=w1000:errorcluster, "VISA resource name out"=w999:refnum<visa-resource-name>)  [unwired: 4 in, 1 out]
          }
        }
        n565 = flat-sequence {
          tunnel: [w989] -> w976
          tunnel: [w990] -> w975
          tunnel: w978 -> [w987]
          tunnel: w977 -> [w988]
          frame #0 {
            n566 = call "Applied Send Command.vi"("error in (no error)"=w988, "Command"=T1."Stop", "VISA resource name"=w987) -> ("error out"=w990:errorcluster, "VISA resource name out"=w989:refnum<visa-resource-name>)  [unwired: 4 in, 1 out]
          }
        }
      }
      event "Reset": Mouse Down {
        n567 = event-data() -> ()  [unwired: 1 in, 7 out]
        n568 = flat-sequence {
          tunnel: [w1021] -> w1007
          tunnel: w1008 -> [w1023]
          tunnel: [w1022] -> w1006
          tunnel: w1009 -> [w1024]
          frame #0 {
            n569 = property on="Reset X Motor Steps" class="DigNum (strict)"() -> ("Value"=w1027:i32)  [unwired: 2 in, 2 out]
            n570 = Number To Decimal String(number=w1027) -> (decimal integer string=w1025:string)  [unwired: 1 in]
            n571 = call "Applied Send Command.vi"("error in (no error)"=w1023, "Extra"=w1025, "Command"=T1."Set ABS Position", "VISA resource name"=w1024) -> ("error out"=w1022:errorcluster, "VISA resource name out"=w1021:refnum<visa-resource-name>)  [unwired: 3 in, 1 out]
          }
        }
        n572 = flat-sequence {
          tunnel: w1013 -> [w1032]
          tunnel: w1012 -> [w1029]
          tunnel: [w1031] -> w1011
          tunnel: [w1030] -> w1010
          frame #0 {
            n573 = property on="Reset Y Motor Steps" class="DigNum (strict)"() -> ("Value"=w1034:i32)  [unwired: 2 in, 2 out]
            n574 = Number To Decimal String(number=w1034) -> (decimal integer string=w1033:string)  [unwired: 1 in]
            n575 = call "Applied Send Command.vi"("error in (no error)"=w1029, "Extra"=w1033, "Command"=T1."Set ABS Position", "VISA resource name"=w1032) -> ("error out"=w1030:errorcluster, "VISA resource name out"=w1031:refnum<visa-resource-name>)  [unwired: 3 in, 1 out]
          }
        }
        n576 = flat-sequence {
          tunnel: [w1019] -> w1003
          tunnel: [w1018] -> w1002
          tunnel: w1005 -> [w1016]
          tunnel: w1004 -> [w1017]
          frame #0 {
            n577 = property on="Reset Z Motor Steps" class="DigNum (strict)"() -> ("Value"=w1020:i32)  [unwired: 2 in, 2 out]
            n578 = Number To Decimal String(number=w1020) -> (decimal integer string=w1014:string)  [unwired: 1 in]
            n579 = call "Applied Send Command.vi"("error in (no error)"=w1017, "Extra"=w1014, "Command"=T1."Set ABS Position", "VISA resource name"=w1016) -> ("error out"=w1018:errorcluster, "VISA resource name out"=w1019:refnum<visa-resource-name>)  [unwired: 3 in, 1 out]
          }
        }
      }
    }
    n580 = flat-sequence {
      frame #0 {
        w648 = 10 ("number of samples")
        n581 = Build Array("GFS") -> (w647:bool[])
        n582 = Boolean To (0,1)(Boolean="GFS") -> (0, 1=w645:i16)
        n583 = call "DAQ AI0"("number of samples"=w648) -> ("data"=w653:dynamicdata)  [unwired: 16 in, 2 out]
        n584 = Multiply(x=w645, y=i16 5) -> (x*y=w643:i16)
        n585 = call "DAQ P1.7"("data"=w647) -> ()  [unwired: 17 in, 2 out]
        n586 = call "Convert from Dynamic Data2"("Dynamic Data Type"=w653) -> ("Array"=w654:dbl[])  [unwired: 3 in]
        n587 = Add Array Elements(numeric array=w654) -> (sum=w652:dbl)
        n588 = Divide(x=w652, y=w648) -> (x/y=w651:dbl)
        n589 = Multiply(x=w643, y=0.8) -> (x*y=w649:dbl)
        n590 = Absolute Value(x=w651) -> (abs(x)=w655:dbl)
        "Dev5 Voltage 2" <- w655
        n591 = Greater?(x=w655, y=w649) -> (0:w656:bool)
        n592 = case shown="True" "Crash Override" {
          tunnel: [w659 TRUE] -> w657
          tunnel: w656 -> [w659 _]
          frame False {
          }
          frame True {
          }
        }
        "Isolated from GND?" <- w657
      }
    }
  }
  n593 = flat-sequence {
    tunnel: w37 -> [w1036]
    tunnel: w36 -> [w1035]
    tunnel: [w1047] -> w21
    frame #0 {
      # "GET CURRENT POSITION"
      n594 = call "Applied Send Command.vi"("error in (no error)"=w1035, "Extra"="", "Command"=T1."Immediate Position?", "VISA resource name"=w1036) -> ("error out"=w1037:errorcluster, "read buffer"=w1042:string, "VISA resource name out"=w1038:refnum<visa-resource-name>)  [unwired: 3 in]
      n595 = call "Applied Send Command.vi"("error in (no error)"=w1037, "Command"=T1."Stop & Kill Buffer", "VISA resource name"=w1038) -> ("error out"=w1044:errorcluster, "VISA resource name out"=w1045:refnum<visa-resource-name>)  [unwired: 4 in, 1 out]
      n596 = Hexadecimal String To Number(string=w1042, offset=3) -> (number=w1039:u32)  [unwired: 1 in, 1 out]
      n597 = VISA Close(VISA resource name=w1045, error in (no error)=w1044) -> ()  [unwired: 1 out]
      n598 = To Long Integer(number=w1039) -> (32bit integer=w1047:i32)
    }
  }
  n599 = flat-sequence {
    tunnel: w23 -> [w1050]
    tunnel: w22 -> [w1049]
    tunnel: [w1048] -> w20
    frame #0 {
      # "GET CURRENT POSITION"
      n600 = call "Applied Send Command.vi"("error in (no error)"=w1049, "Extra"="", "Command"=T1."Immediate Position?", "VISA resource name"=w1050) -> ("error out"=w1051:errorcluster, "read buffer"=w1056:string, "VISA resource name out"=w1052:refnum<visa-resource-name>)  [unwired: 3 in]
      n601 = call "Applied Send Command.vi"("error in (no error)"=w1051, "Command"=T1."Stop & Kill Buffer", "VISA resource name"=w1052) -> ("error out"=w1058:errorcluster, "VISA resource name out"=w1059:refnum<visa-resource-name>)  [unwired: 4 in, 1 out]
      n602 = Hexadecimal String To Number(string=w1056, offset=3) -> (number=w1053:u32)  [unwired: 1 in, 1 out]
      n603 = VISA Close(VISA resource name=w1059, error in (no error)=w1058) -> ()  [unwired: 1 out]
      n604 = To Long Integer(number=w1053) -> (32bit integer=w1048:i32)
    }
  }
  n605 = flat-sequence {
    tunnel: w25 -> [w1062]
    tunnel: w24 -> [w1061]
    tunnel: [w1063] -> w19
    frame #0 {
      # "GET CURRENT POSITION"
      n606 = call "Applied Send Command.vi"("error in (no error)"=w1061, "Extra"="", "Command"=T1."Immediate Position?", "VISA resource name"=w1062) -> ("error out"=w1064:errorcluster, "read buffer"=w1069:string, "VISA resource name out"=w1065:refnum<visa-resource-name>)  [unwired: 3 in]
      n607 = call "Applied Send Command.vi"("error in (no error)"=w1064, "Command"=T1."Stop & Kill Buffer", "VISA resource name"=w1065) -> ("error out"=w1071:errorcluster, "VISA resource name out"=w1072:refnum<visa-resource-name>)  [unwired: 4 in, 1 out]
      n608 = Hexadecimal String To Number(string=w1069, offset=3) -> (number=w1066:u32)  [unwired: 1 in, 1 out]
      n609 = VISA Close(VISA resource name=w1072, error in (no error)=w1071) -> ()  [unwired: 1 out]
      n610 = To Long Integer(number=w1066) -> (32bit integer=w1063:i32)
    }
  }
  n611 = flat-sequence {
    tunnel: w21 -> [w1078]
    tunnel: w20 -> [w1077]
    tunnel: w19 -> [w1076]
    frame #0 {
      n612 = Build Array(w1078, w1077, w1076) -> (w1074:i32[])
      n613 = call-poly <vilib>:"Write To Spreadsheet File.vi"("1D data"=w1074, "file path (dialog if empty)"=path "S:/SSE/SCL2/POS.TXT") -> ()  [unwired: 6 in, 1 out]
    }
    frame #1 {
    }
  }
